vi "SHG_polarization_resolved.vi"() -> ()   [LabVIEW 2022 SP3]
uses:
  PMT_VIs/Logo.ctl
  C:/Users/Public/OneDrive/Desktop/PMT_Project_folder/Kinesis_VIs/Thorlabs.MotionControl.Controls.dll
  Kinesis_VIs/Thorlabs.MotionControl.Controls.dll
  <vilib>/Utility/file.llb/Write Delimited Spreadsheet (string).vi
  <vilib>/Utility/file.llb/Write Delimited Spreadsheet (I64).vi
  <vilib>/Utility/file.llb/Write Delimited Spreadsheet (DBL).vi
  C:/Users/Public/OneDrive/Desktop/PMT_Project_folder/Kinesis_VIs/ThorLabs.MotionControl.KCube.DCServoCLI.dll
  Kinesis_VIs/ThorLabs.MotionControl.KCube.DCServoCLI.dll
  <vilib>/Analysis/NI_AALBase.lvlib
panel:
  in  "Rotating":dbl(ring)=2.0 items=["Analyzer"=1.0, "Polarizer"=2.0, ""=0.0]
  in  "Analyzer config":string="165"
  in  "Polarizer config":string=" rotate"
  in  "autosweep file to save":path=path "D:/LabData/XiaoWang_Group_data_2024on/StackingTransitions/NbOI2/Lvgroup/samples/22p5deg/SHG/flake2_pos1_analyzer-y.txt"
  in  "SP 2":dbl=-5.0 caption="Second Polarizer Start Position \n Set"
  out "SPD 2":dbl=-5.0 caption="Analyzer Start Position Read"
  in  "second motor T/F":bool
  out "PC 2":dbl caption="Second Polarizer Current Position"
  in  "Motor Controller\nSerialNumber 2":string="27261255"
  in  "KCubeDCServoControl 2":refnum<k24>(container)
  out "Polar Plot":picture
  in  "Wait to Start (ms)":i32
  in  "Laser Power (mW)":string="3"
  in  "Sample Name":string="NbOI2 22.5deg flake2 pos1 analyzer-y"
  in  "Save All Gate Data":bool
  out "ESD":dbl caption="Steps\nAdded/Removed"
  in  "ES":dbl caption="Add /Remove \nSteps"
  out "Sweep Graph":u32[](graph)=[236, 252, 257, 253, 238, 214, 204, 173, 152, 146, 141, 143, 145, 162, 179, 184, 196, 197, 202, 190, 177, 161, 155, 148, 142, 151, 152, 169, 188, 216, 224, 233, 239, 236, 224, 211, 194, 170, 151, 147, 143, 143, 157, 168, 177, 196, 198, 205, 196, 190, 170, 163, 146, 136, 133, 134, 144, 165, 186, 211, 229]
  out "SM":i32 caption="Sweep\nMean"
  out "SN":i32=61 caption="Current Sweep Iteration"
  out "SND":i32=61 caption="Total No. of Sweeps"
  in  "Auto-Sweep":bool
  in  "P8":bool
  out "PC":dbl caption="Current Position"
  out "WTD":i32=2500 caption="Wait Time \n(ms) Read"
  out "EPD":dbl=183.0 caption="End Position\nRead"
  out "SPD":dbl caption="Start Position\nRead"
  out "SSD":dbl=3.0 caption="Step Size\nRead"
  in  "SP":dbl caption="Start Position Set"
  in  "WT":i32=2500 caption="Wait Time (ms)\n Set"
  in  "EP":dbl=183.0 caption="End Position Set"
  in  "P7":bool
  in  "SS":dbl=3.0 caption="Step Size Set"
  in  "Motor Controller\nSerialNumber":string="27268499"
  in  "KCubeDCServoControl":refnum<k24>(container)
  in  "Export":bool
  out "DB":u32[](array[numeric])=[235, 0, 0, 0, 0, 0, 0, 0, 0, 0, 0, 0, 0, 0, 0, 0]
  out "OVL":bool caption="LED ON : Over Rang Data"
  out "OLD":i32
  out "GN":i32 caption="Gate Number"
  in  "Correction":bool=TRUE
  in  "Logo":T1
  out "Graph":u32[](graph)=[235]
  in  "Stop":bool
  in  "Start":bool
  in  "P6":bool
  out "RND":i32=20 caption="Read Number\nRead Data"
  in  "P5":bool
  in  "RN":i32=20 caption="Read Number\nSet Data"
  out "PowerD":i32=1 caption="Power\nRead Data"
  out "ITD":i32=400 caption="Internal Time\nRead Data"
  in  "P4":bool
  in  "P3":bool
  in  "IT":i32=400 caption="Internal Time\nSet Data"
  in  "P2":bool
  out "Handle Number":i32=172291552
  in  "P1":bool=TRUE caption="Switch\nPower OFF/Power ON"
  in  "EXIT":bool=TRUE
  # "pmt serial: 30430219"
  # "can't change after running. exit to change"
  # "number in degrees."
  # "y-165\nx-75"
  # "y-82.5\nx-37.5"
  # "polarizer: 27268499\nanalyzer: 2726155"
  # "note: If you change angle between linear polarized light and half-wave plate by theta, the \npolarization after the wave plate is changed by twice theta. The code doesn't account for this.\nThis means we really need to go only to 180degrees, because at that point we have rotated the polarization by 360deg."
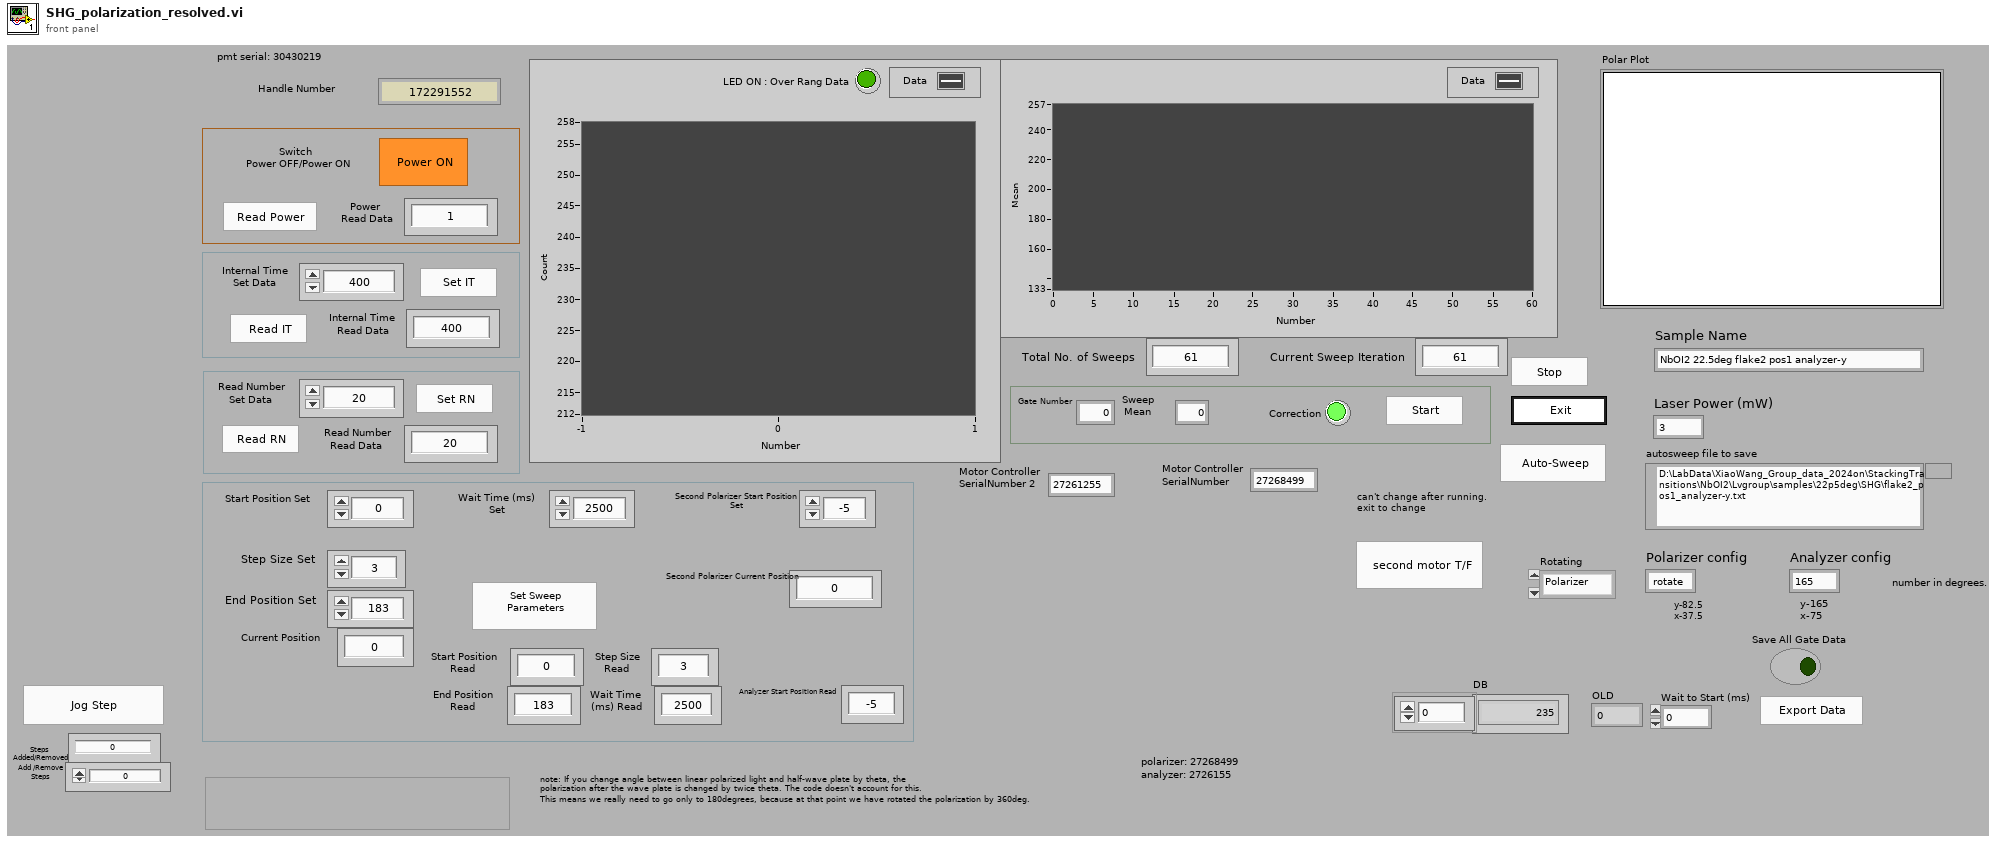
[diagram p1: front panel]
types:
  T1 = typedef "Logo.ctl" = bool
  T2 = enum8{"Enabled", "Disabled", "Disabled and Grayed Out"}
  T3 = typedef "LVBoundsTypeDef.ctl" = cluster{"Width":u32, "Height":u32}
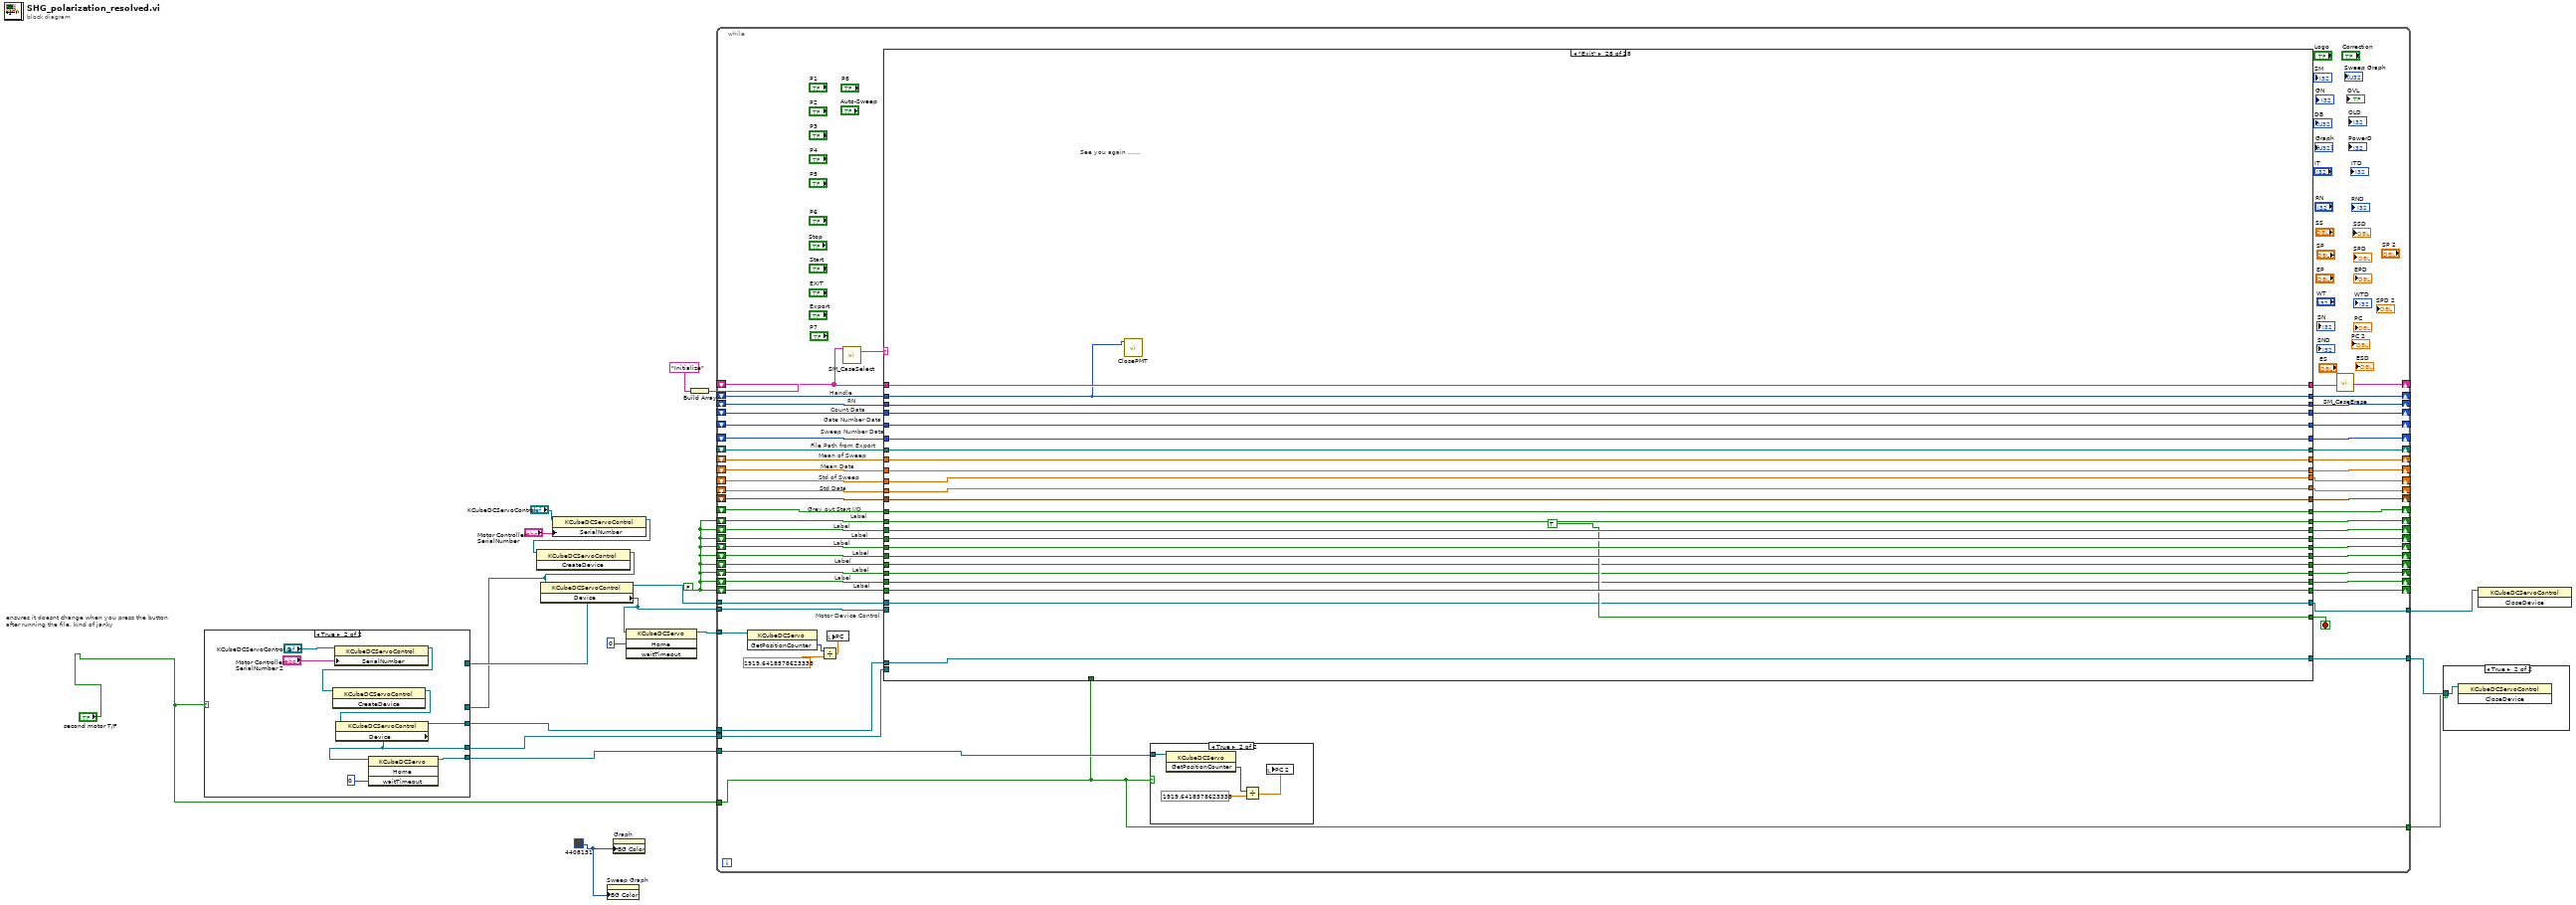
[diagram p0: block diagram]
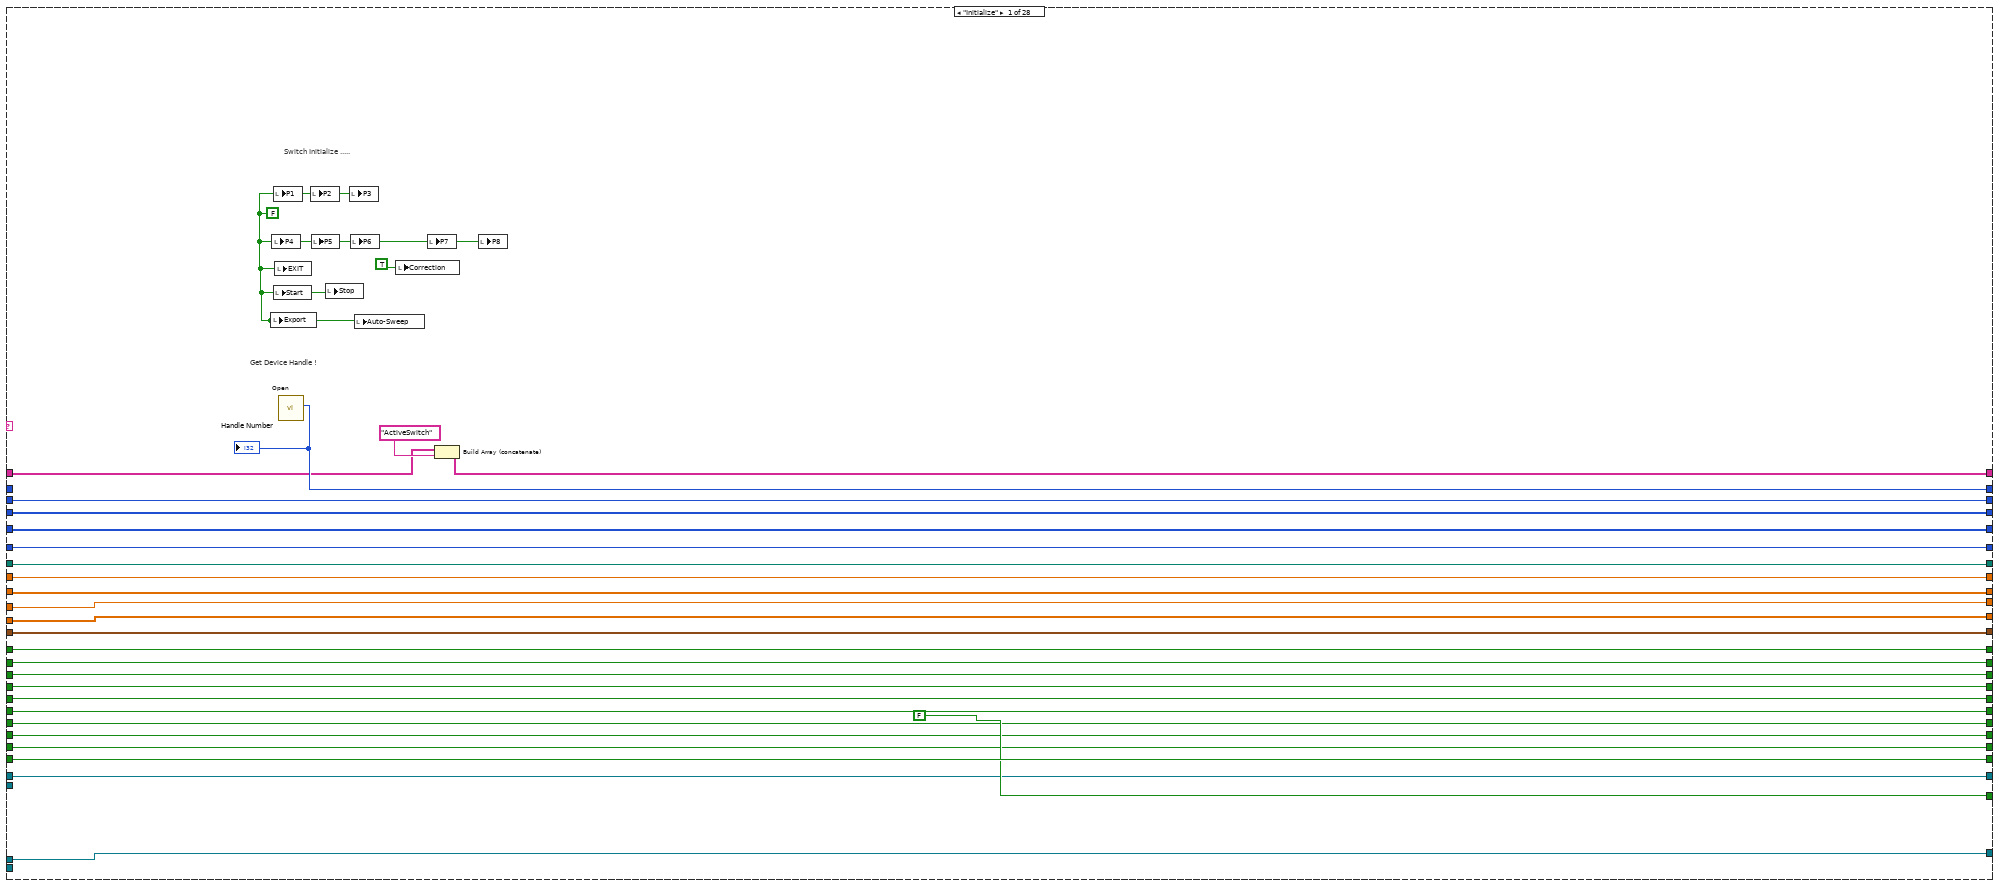
[diagram p5: hidden frame]
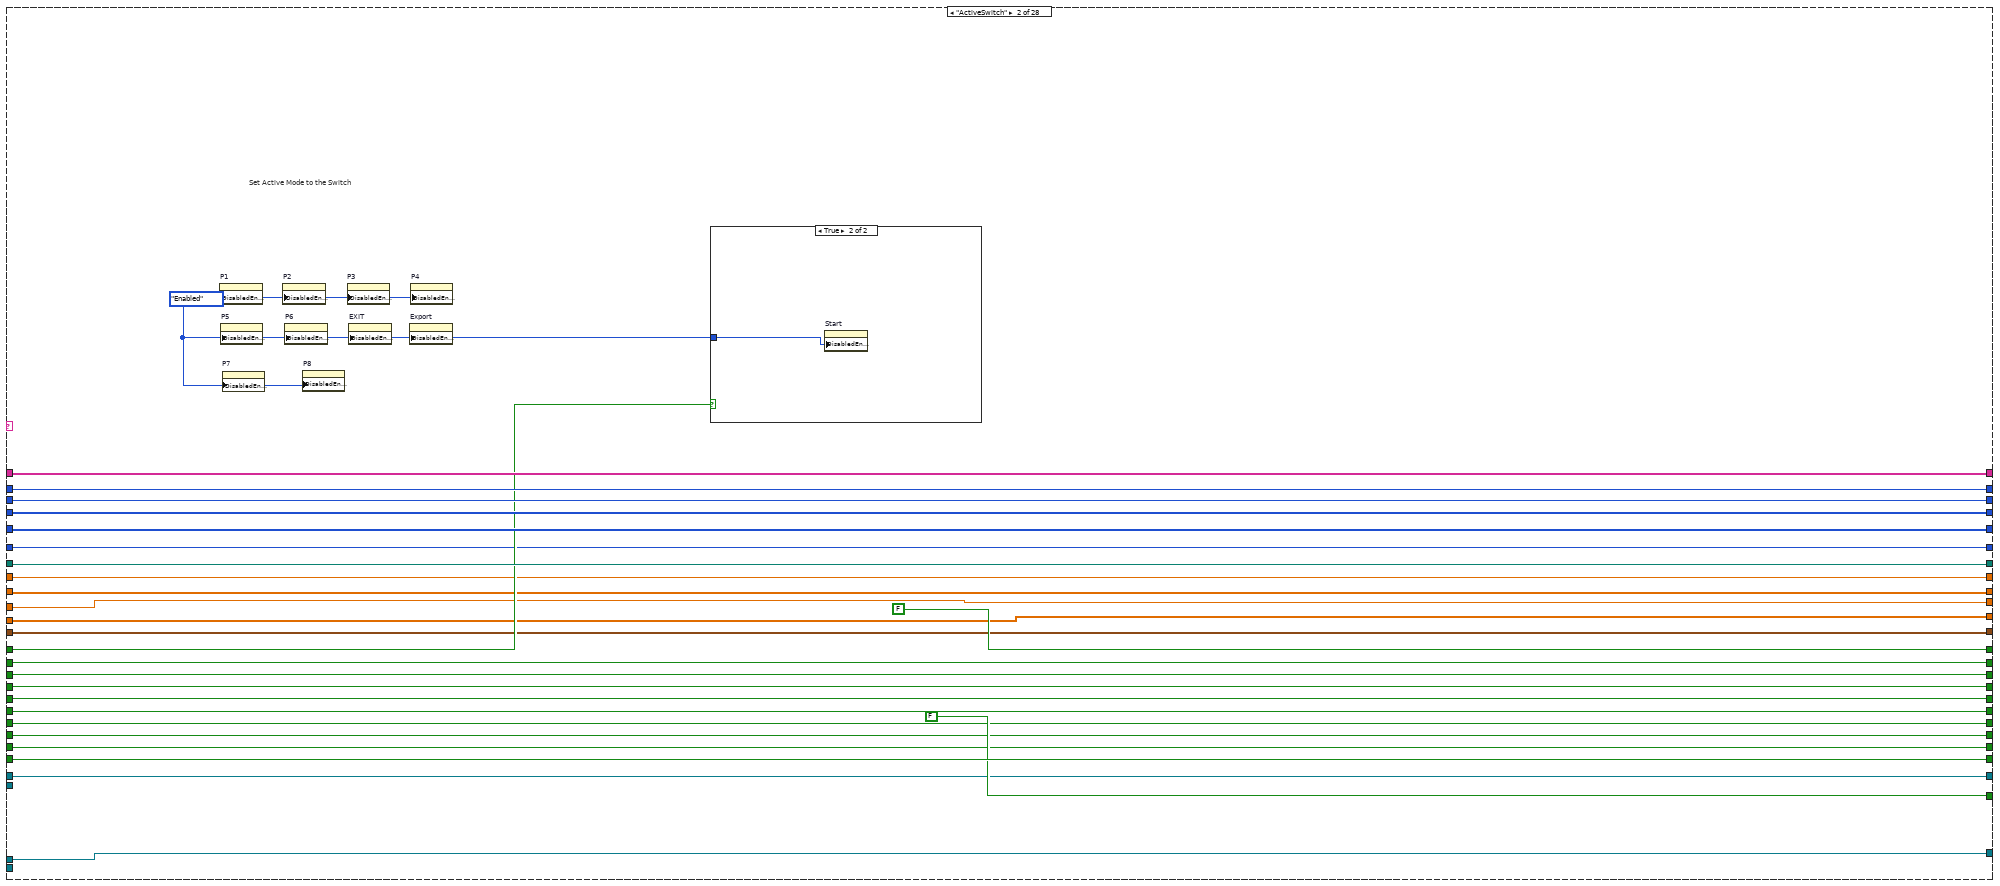
[diagram p6: hidden frame]
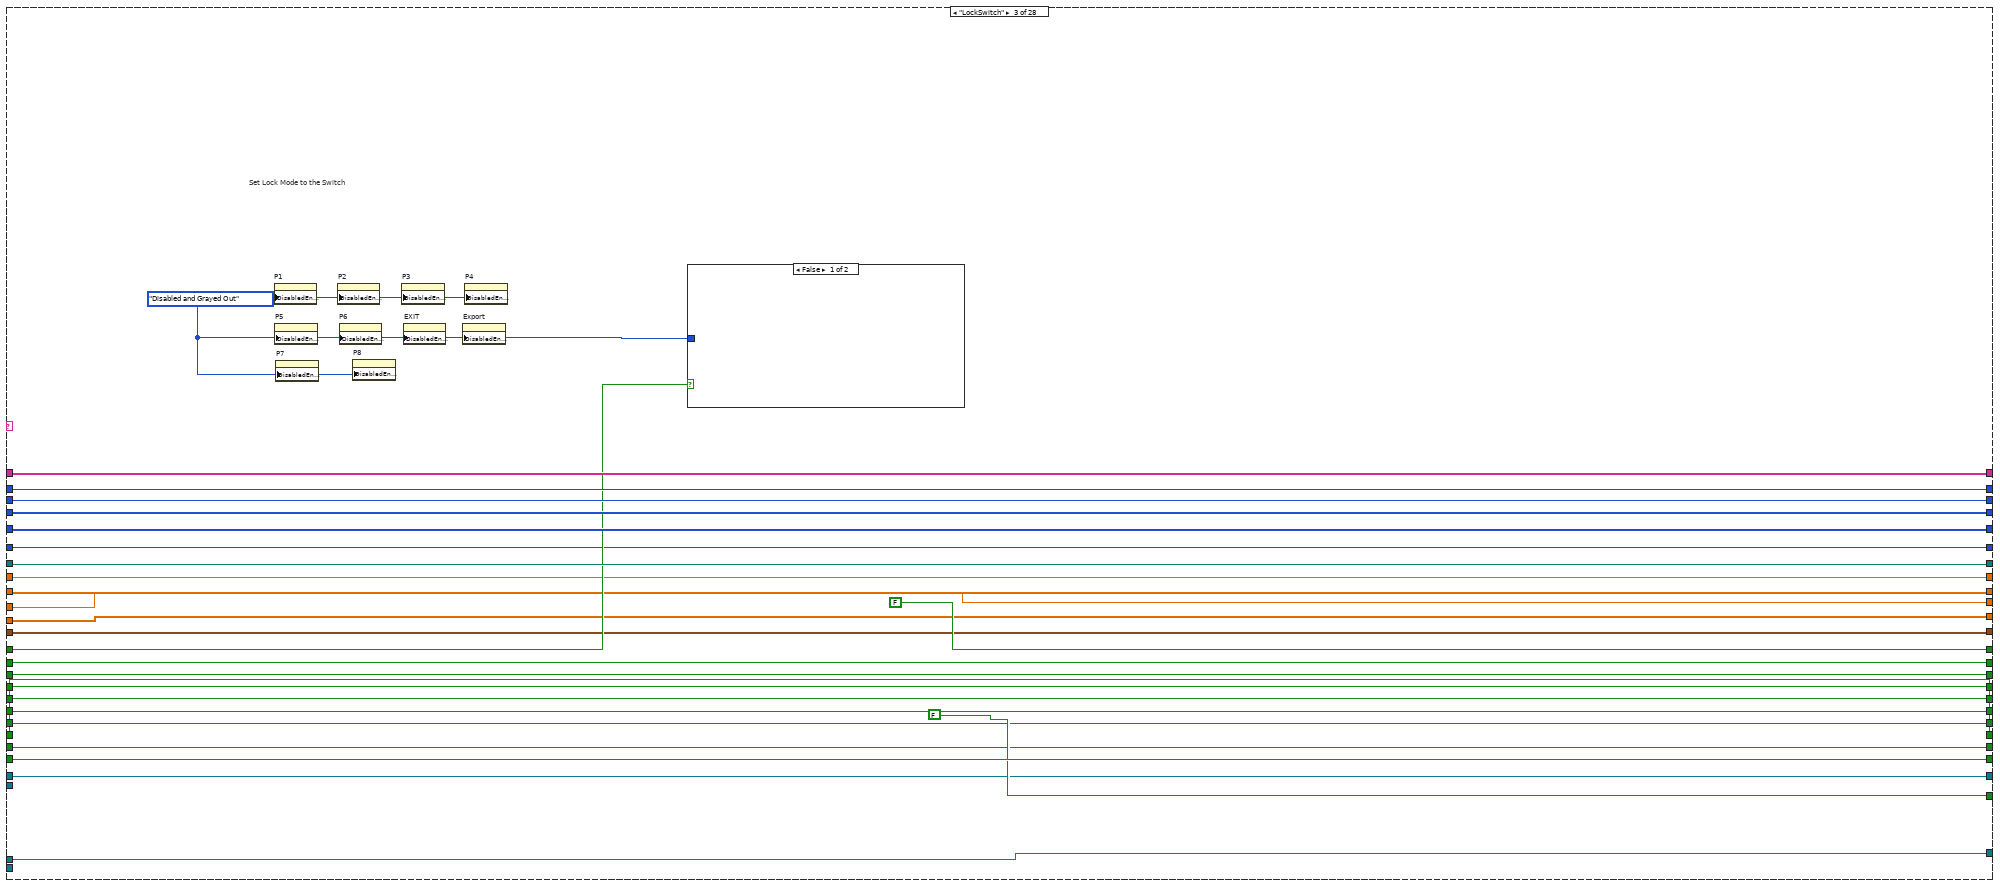
[diagram p8: hidden frame]
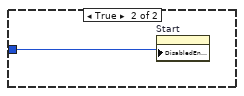
[diagram p9: hidden frame]
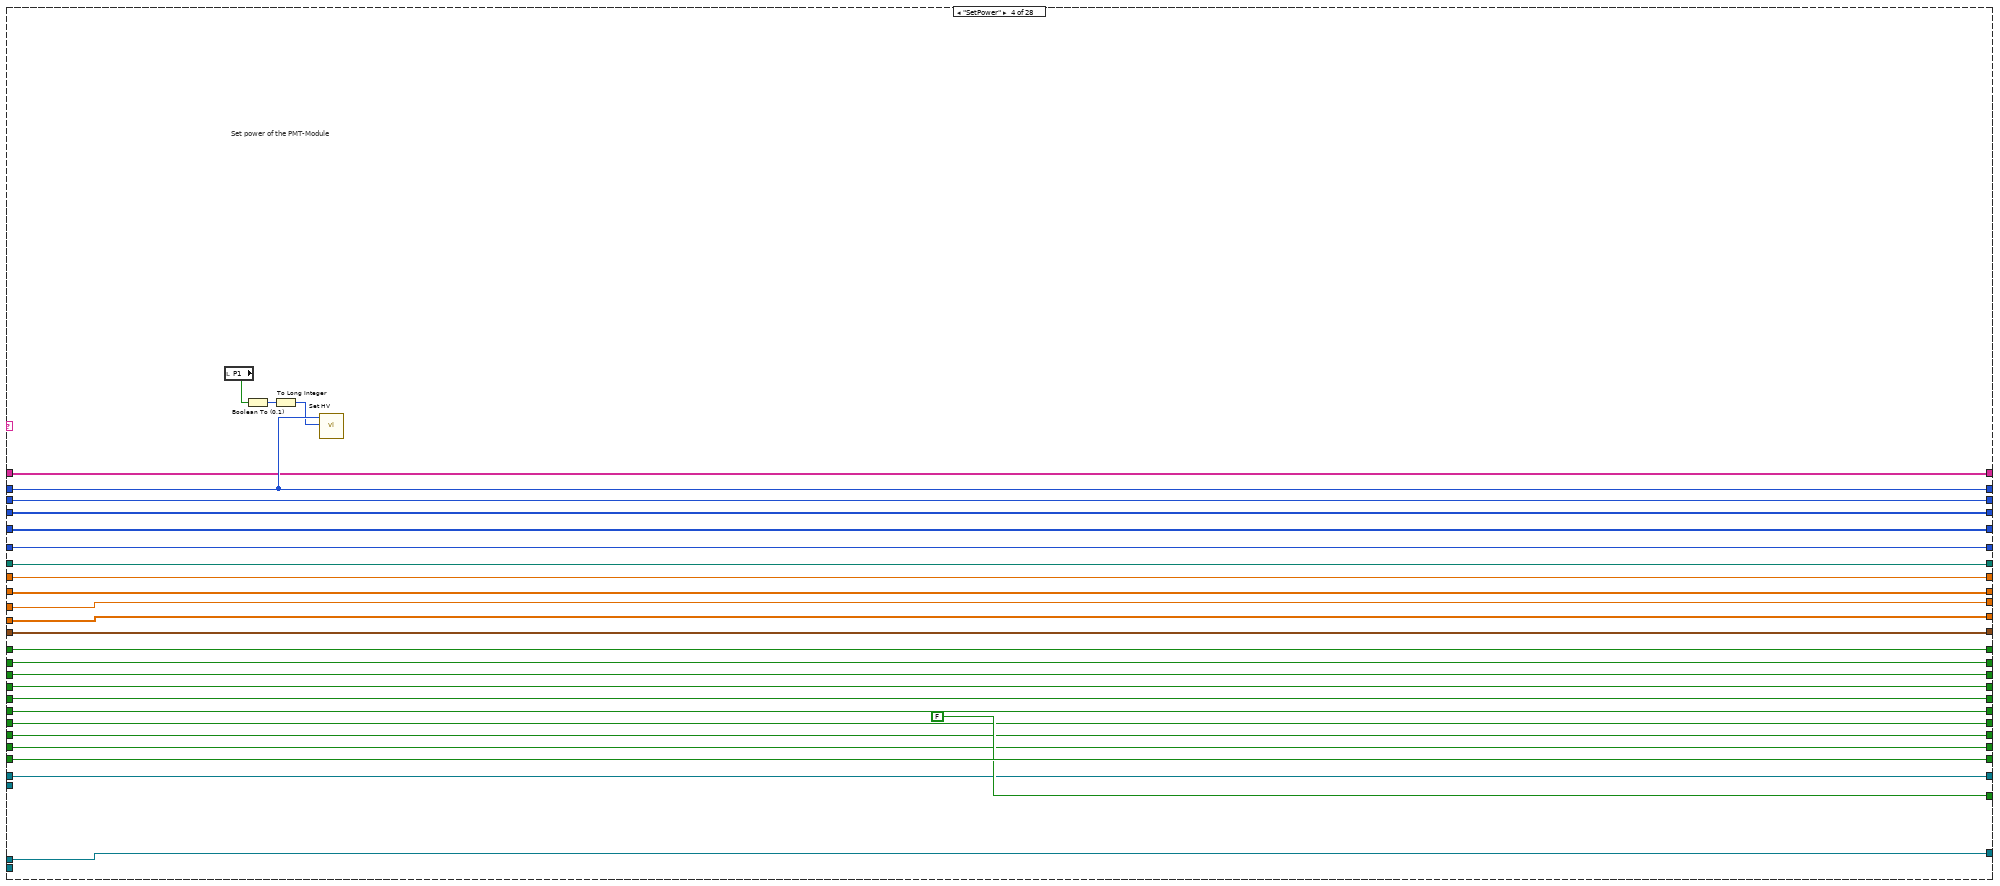
[diagram p10: hidden frame]
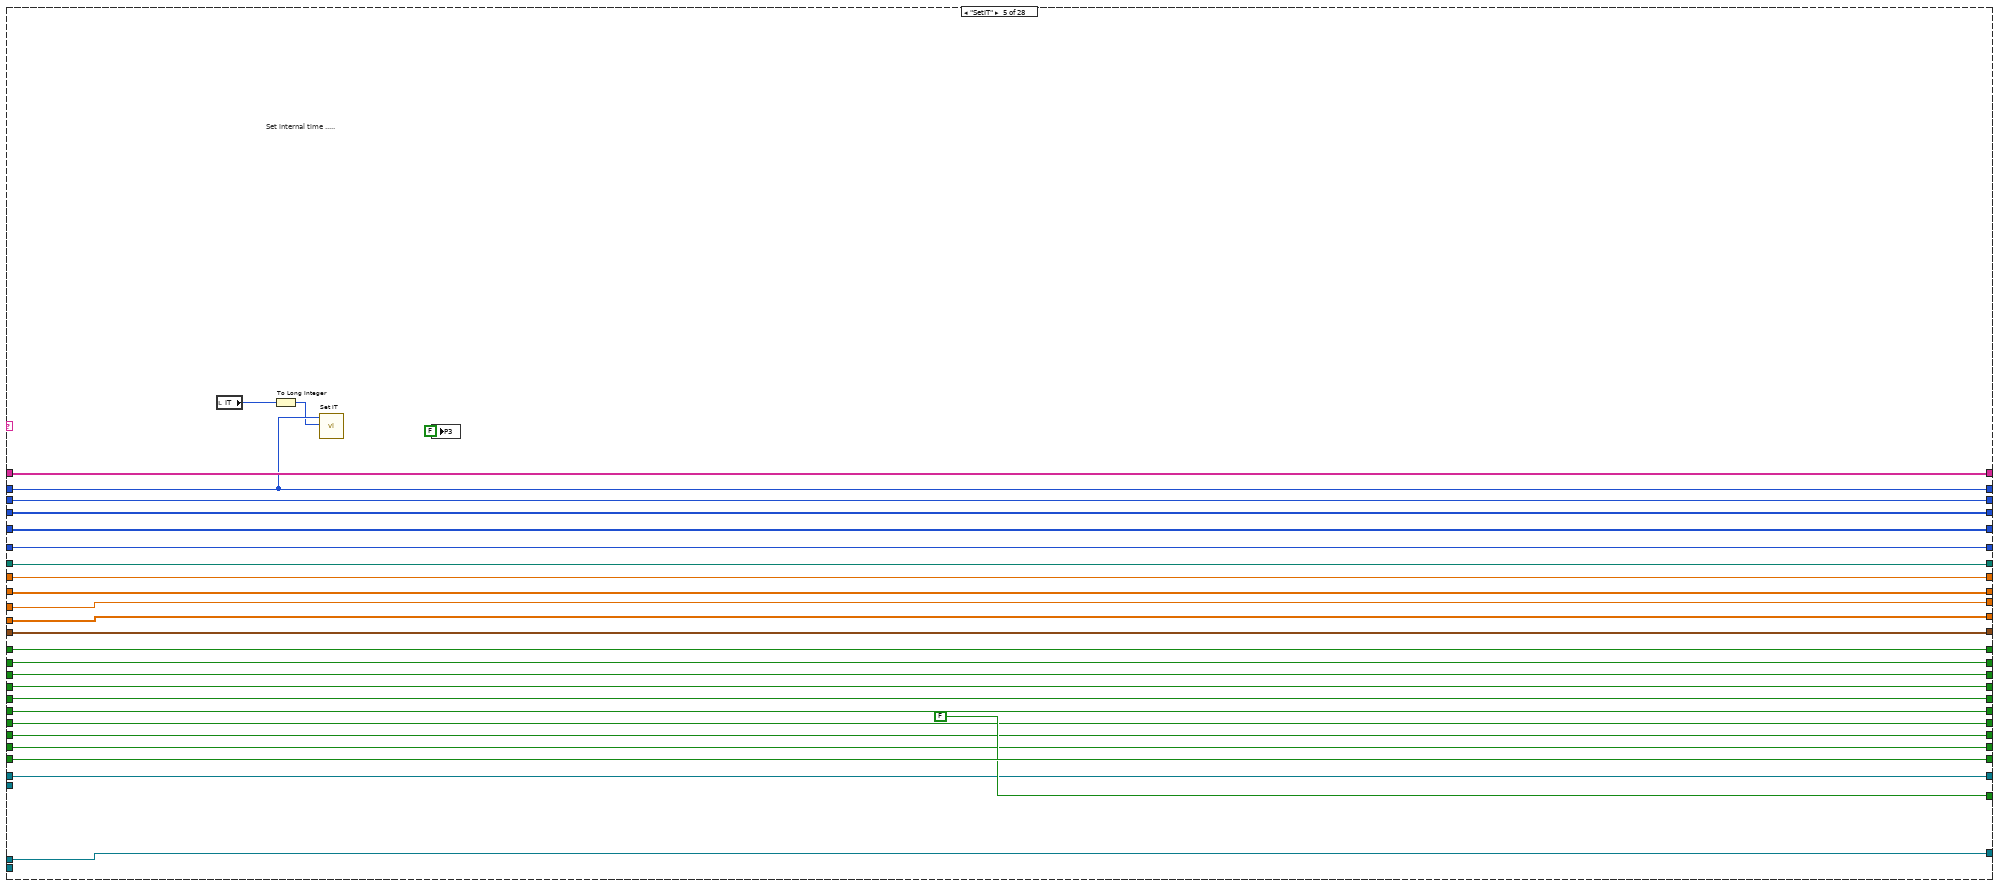
[diagram p11: hidden frame]
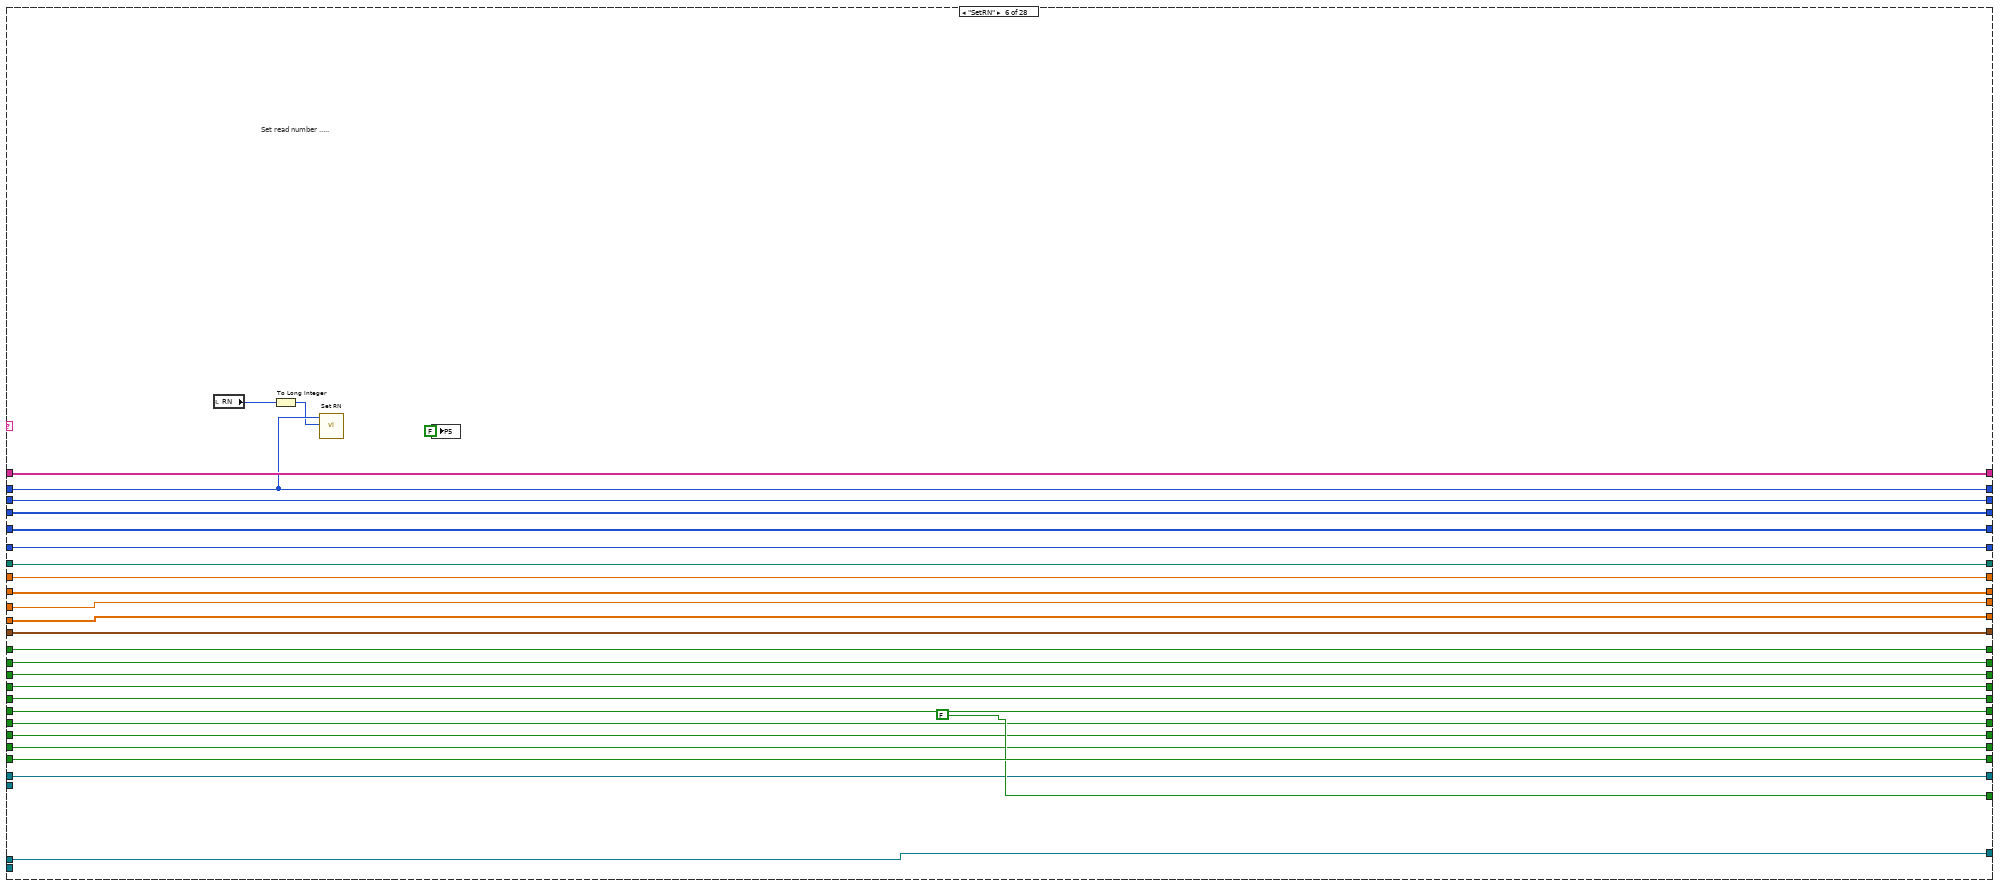
[diagram p12: hidden frame]
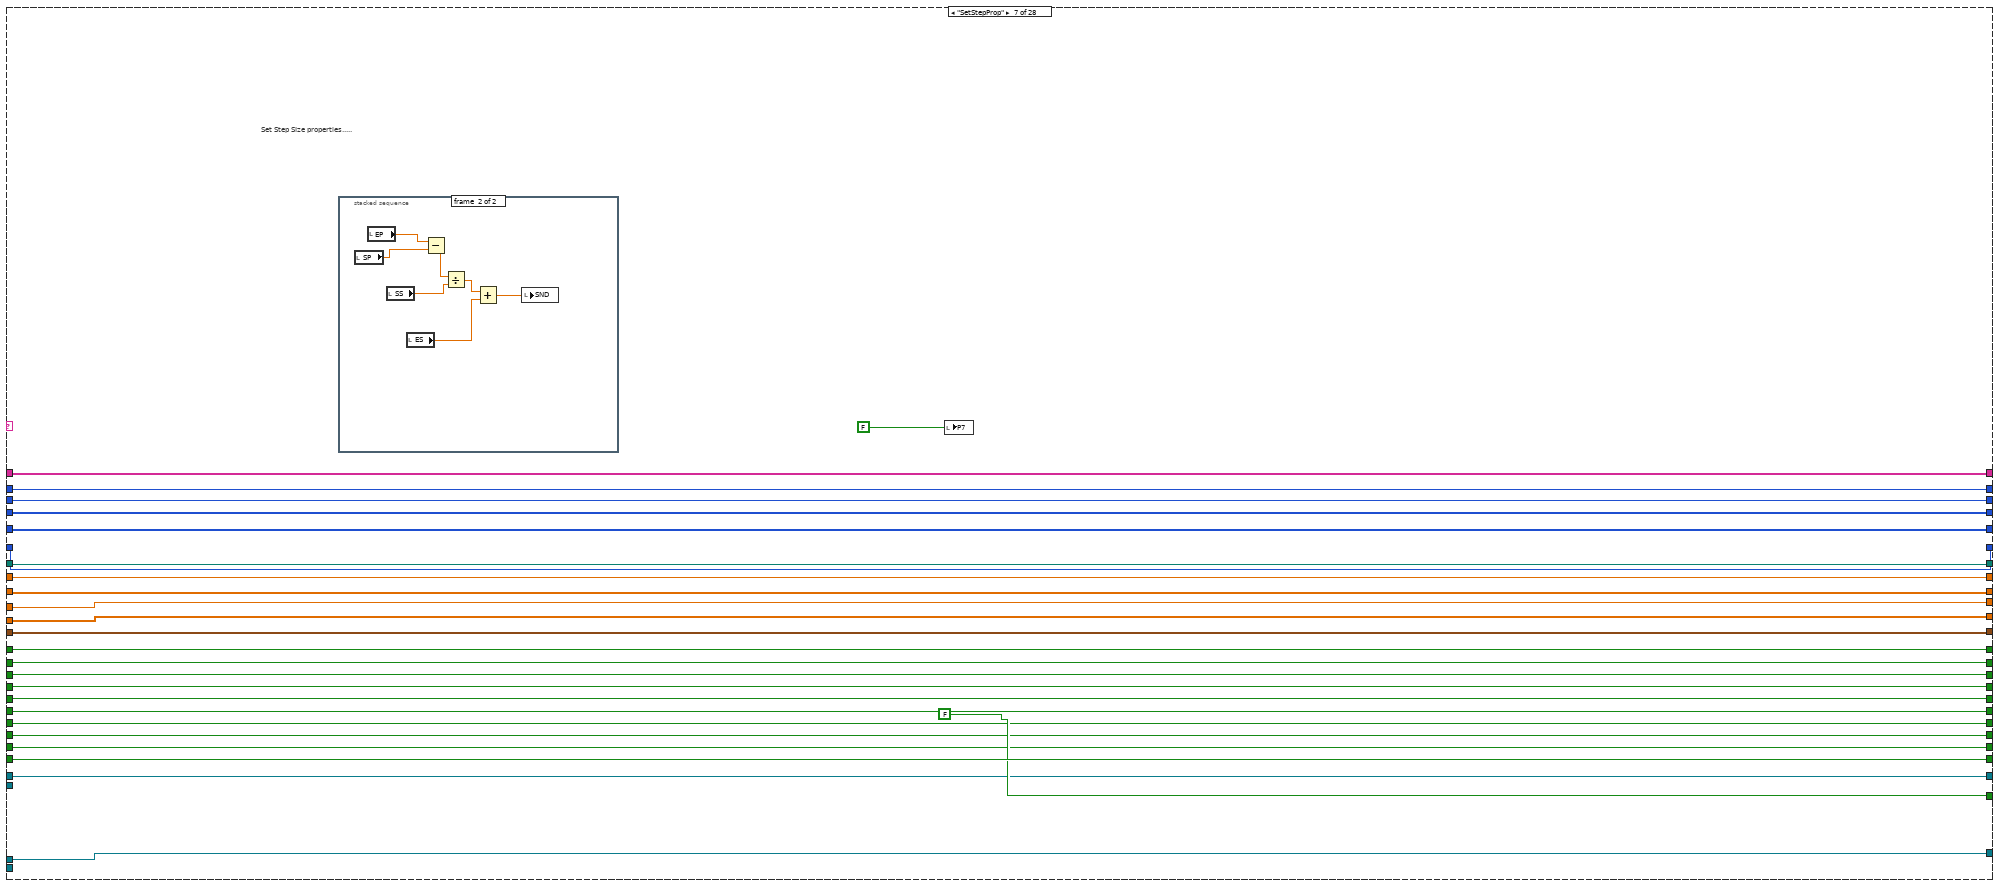
[diagram p13: hidden frame]
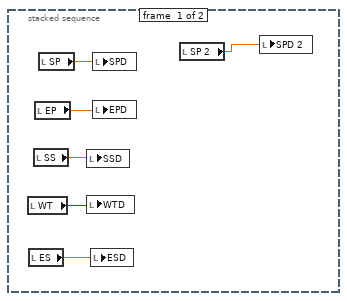
[diagram p14: hidden frame]
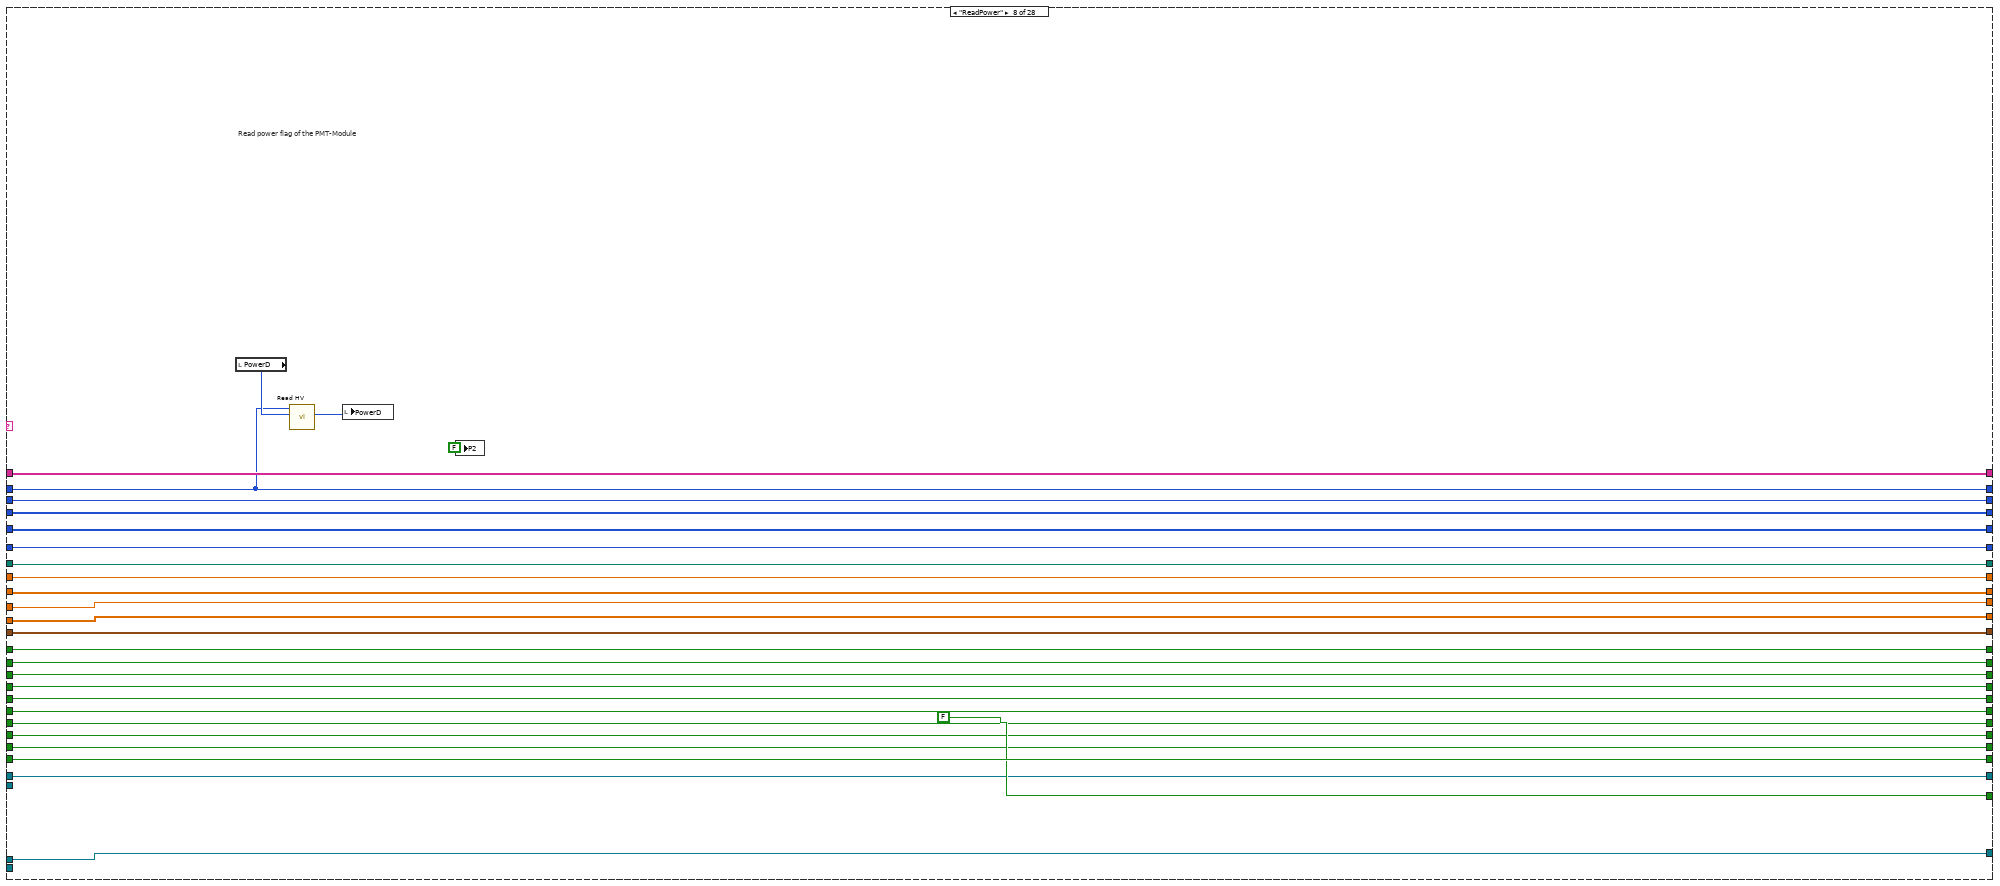
[diagram p15: hidden frame]
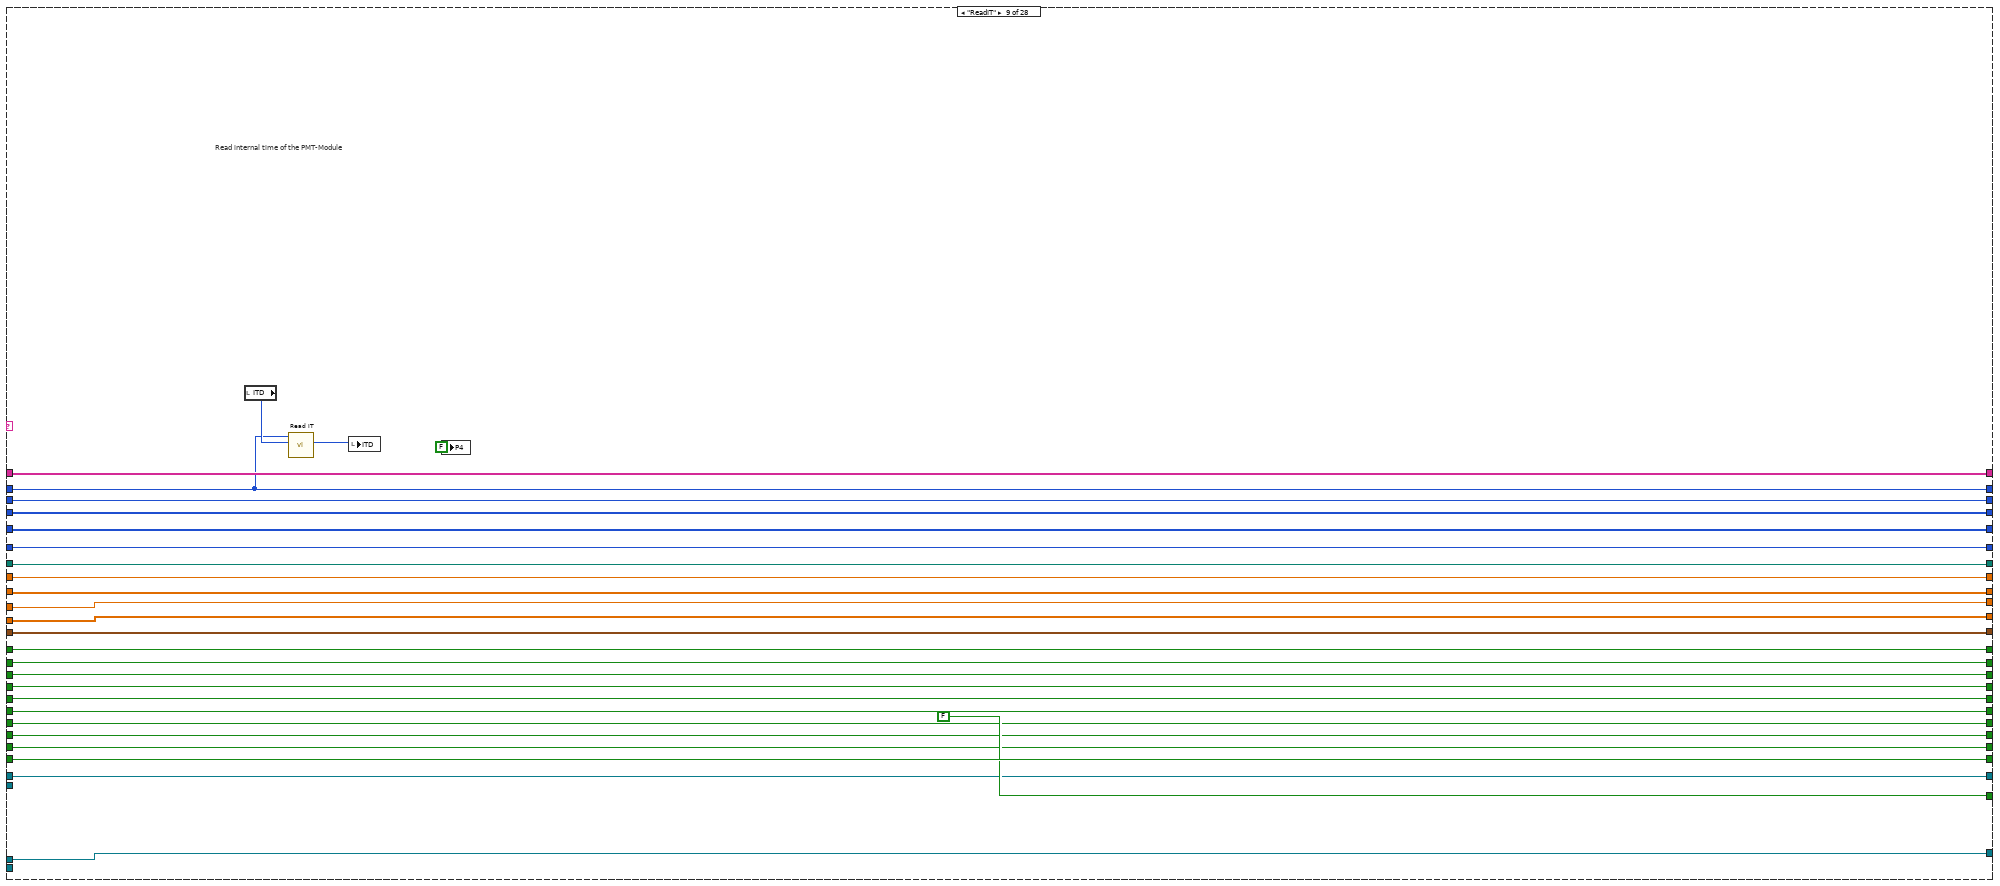
[diagram p16: hidden frame]
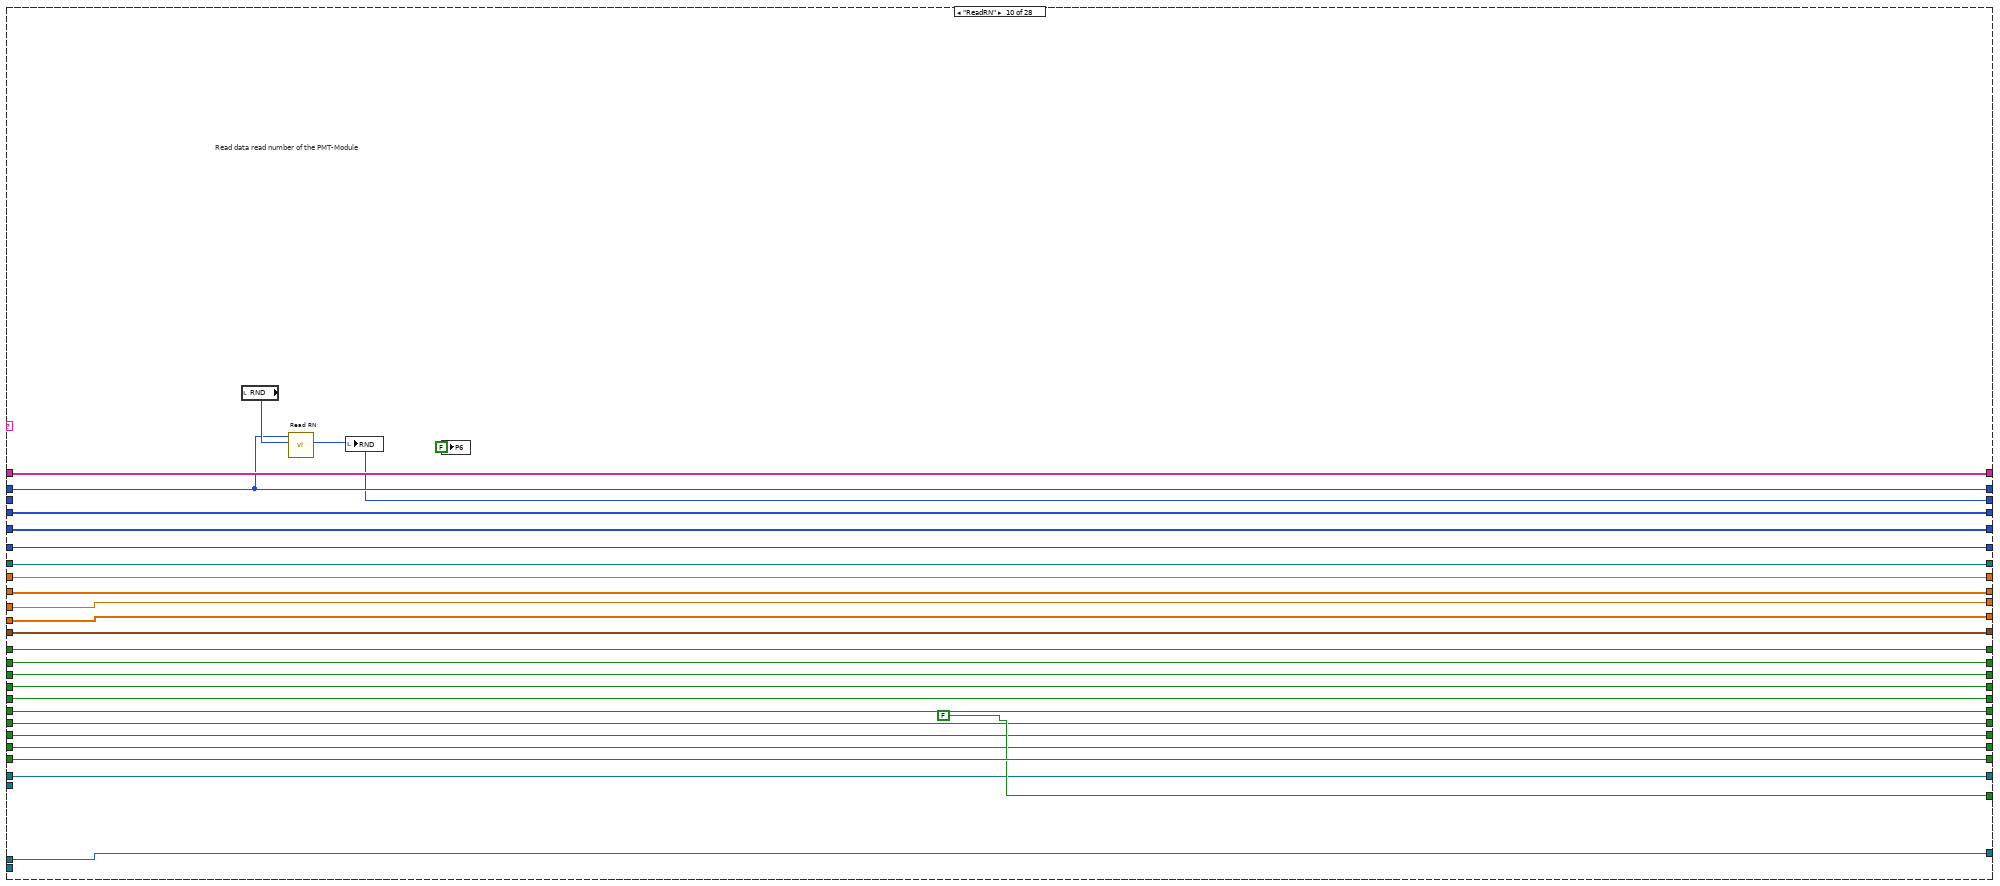
[diagram p17: hidden frame]
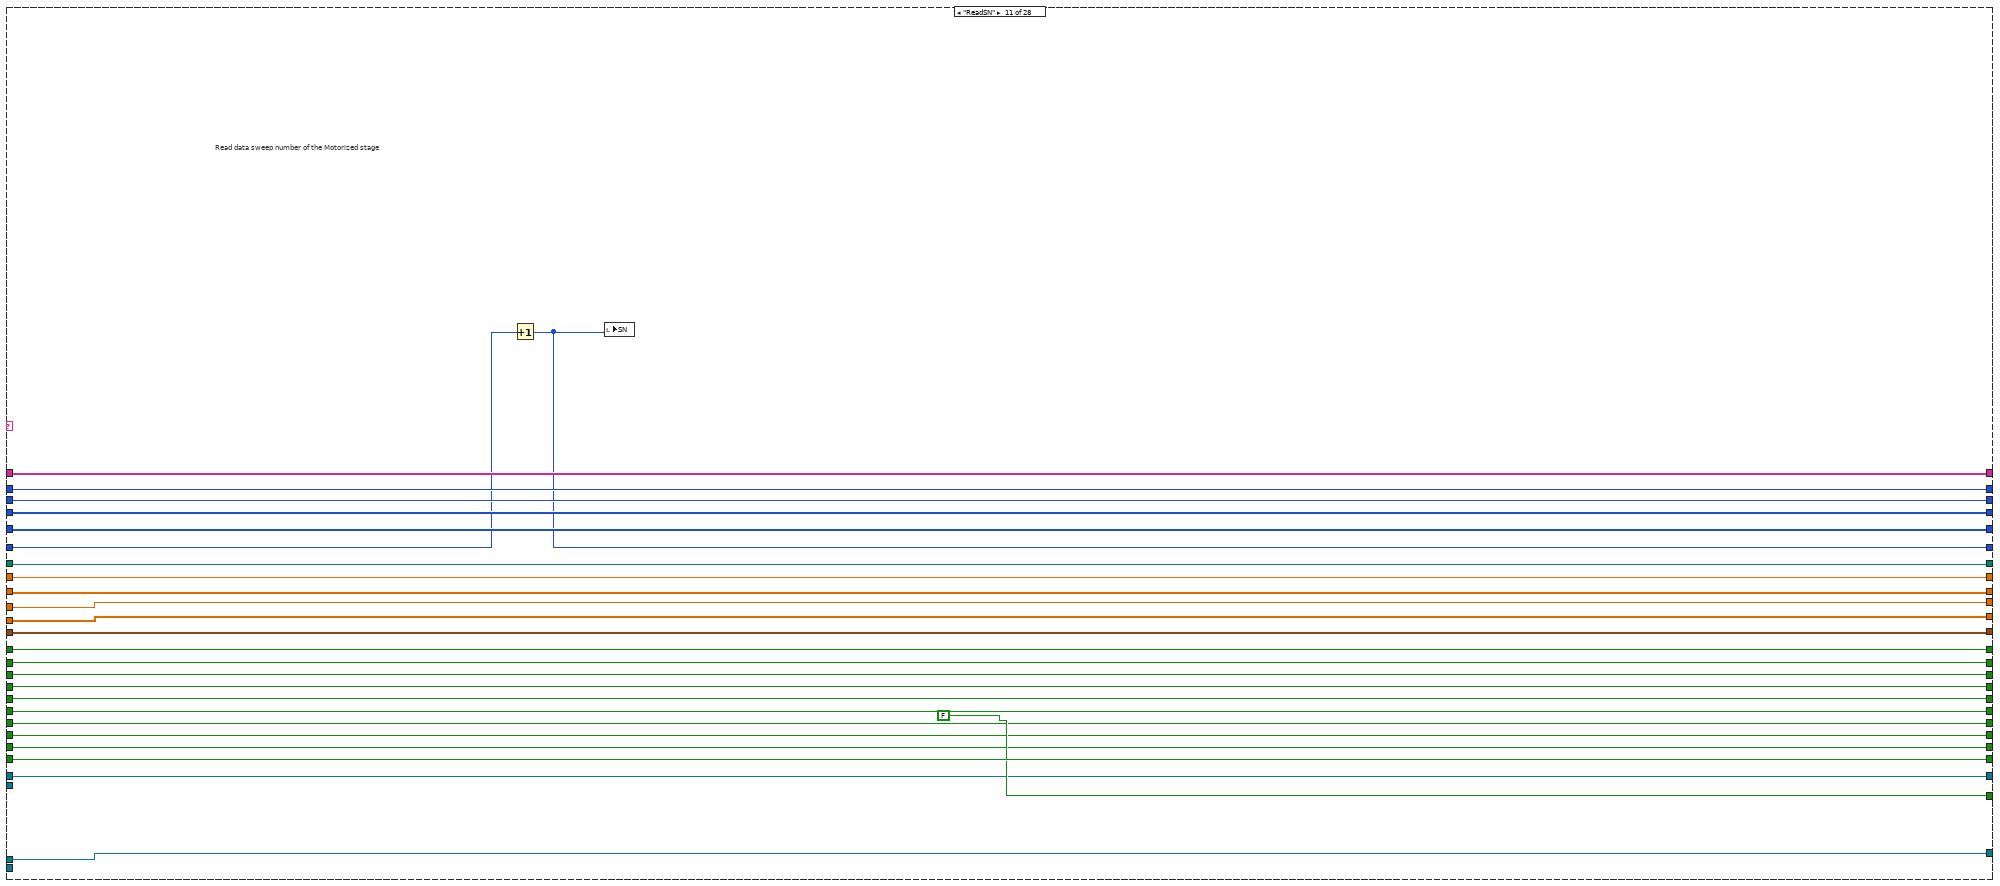
[diagram p18: hidden frame]
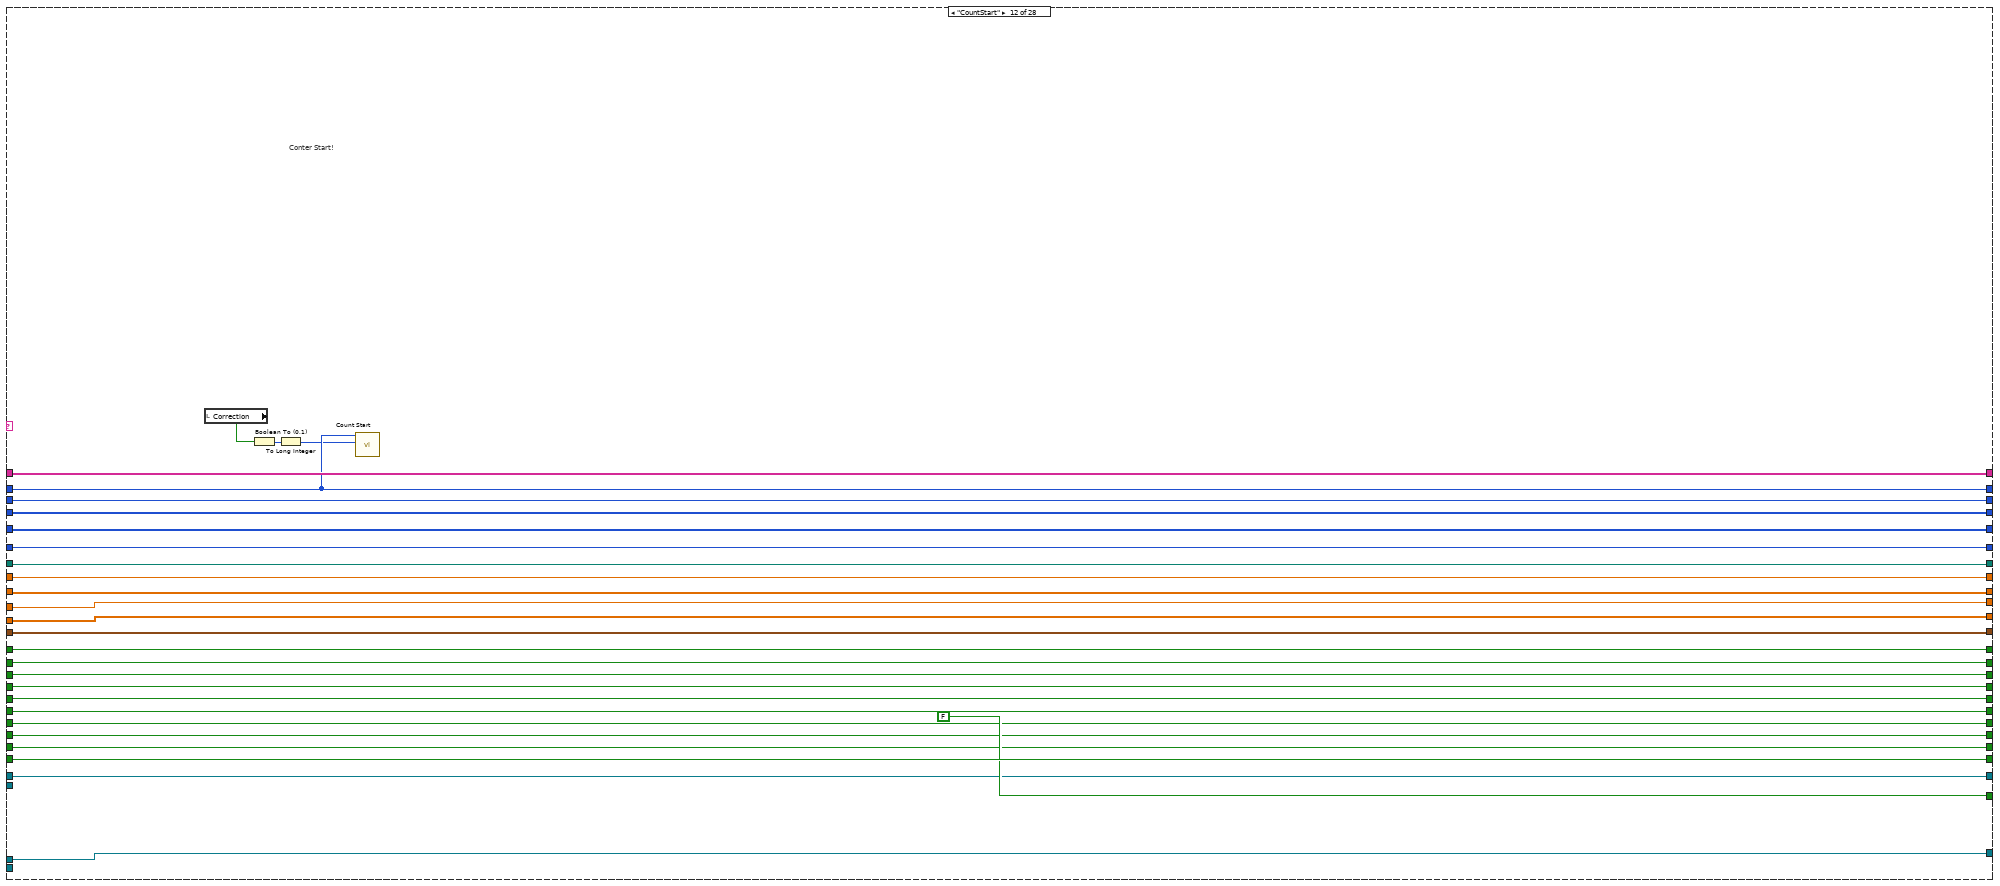
[diagram p19: hidden frame]
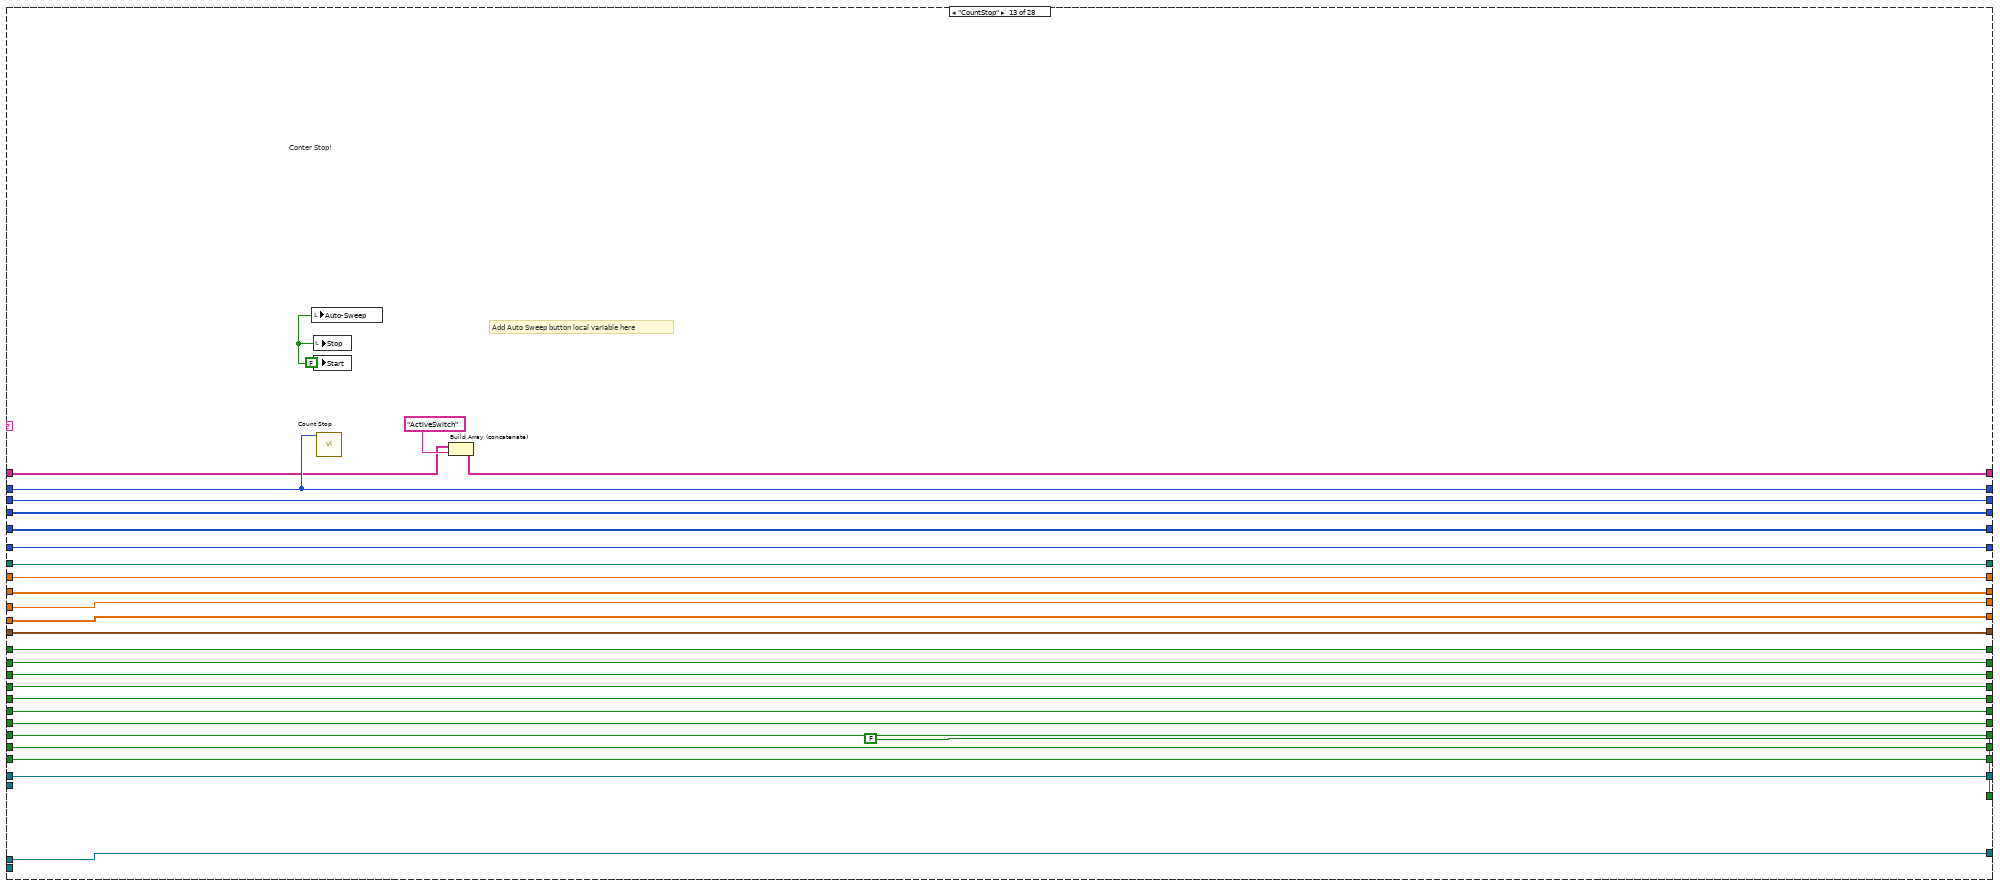
[diagram p20: hidden frame]
diagram:
  w1 = u32 4408131
  w17 = FALSE
  # "ensures it doesnt change when you press the button \nafter running the file. kind of janky"
  n1 = property class="KCubeDCServoControl"(reference="KCubeDCServoControl", "SerialNumber"="Motor Controller\nSerialNumber") -> (reference out=w16:refnum<k24>)  [unwired: 1 in, 1 out]
  n2 = invoke class="KCubeDCServoControl" method="CreateDevice"(reference=w16) -> (reference out=w4:refnum<k24>)  [unwired: 2 in, 2 out]
  n3 = property class="KCubeDCServoControl"(reference=w4) -> (reference out=w13:refnum<k24>, "Device"=w5:refnum<k24>)  [unwired: 1 in, 1 out]
  n4 = case shown="True" "second motor T/F" {
    tunnel: [w20 w24] -> w9
    tunnel: [w20 w23] -> w8
    tunnel: [w21 w22] -> w7
    tunnel: w5 -> [w20 _]
    tunnel: w4 -> [w21 _]
    frame False {
      # "just connect to the first one. it won't be sused"
    }
    frame True {
      n5 = property class="KCubeDCServoControl"(reference="KCubeDCServoControl 2", "SerialNumber"="Motor Controller\nSerialNumber 2") -> (reference out=w29:refnum<k24>)  [unwired: 1 in, 1 out]
      n6 = invoke class="KCubeDCServoControl" method="CreateDevice"(reference=w29) -> (reference out=w26:refnum<k24>)  [unwired: 2 in, 2 out]
      n7 = property class="KCubeDCServoControl"(reference=w26) -> (reference out=w22:refnum<k24>, "Device"=w23:refnum<k24>)  [unwired: 1 in, 1 out]
      n8 = invoke class="KCubeDCServo" method="Home"(reference=w23, "waitTimeout"=0) -> (reference out=w24:refnum<k24>)  [unwired: 2 in, 3 out]
    }
  }
  n9 = property on="Sweep Graph" class="WFGraph (strict)"("BG Color"=w1) -> ()  [unwired: 2 in, 2 out]
  n10 = property on="Graph" class="WFGraph (strict)"("BG Color"=w1) -> ()  [unwired: 2 in, 2 out]
  n11 = invoke class="KCubeDCServo" method="Home"(reference=w5, "waitTimeout"=0) -> (reference out=w11:refnum<k24>)  [unwired: 2 in, 3 out]
  n12 = Build Array("Initialize") -> (w18:string[])
  n13 = while {
    shift-right: [w71] -> _
    shift-left: w17 -> [w72]
    shift-right: [w73] -> _
    shift-left: w17 -> [w74]
    shift-right: [w75] -> _
    shift-left: w17 -> [w76]
    shift-right: [w77] -> _
    shift-left: w17 -> [w78]
    shift-right: [w79] -> _
    shift-left: _ -> [w80]
    shift-right: [w81] -> _
    shift-left: _ -> [w82]
    shift-right: [w83] -> _
    shift-left: _ -> [w84]
    shift-right: [w69] -> _
    shift-left: w17 -> [w70]
    shift-right: [w87] -> _
    shift-left: w17 -> [w88]
    shift-right: [w66] -> _
    shift-left: w18 -> [w85]
    shift-right: [w64] -> _
    shift-left: w17 -> [w65]
    shift-right: [w62] -> _
    shift-left: w17 -> [w63]
    shift-right: [w61] -> _
    shift-left: w17 -> [w60]
    tunnel: w13 -> [w57]
    tunnel: [w56] -> w14
    shift-right: [w59] -> _
    shift-left: _ -> [w58]
    tunnel: w5 -> [w55]
    shift-right: [w54] -> _
    shift-left: _ -> [w53]
    shift-right: [w52] -> _
    shift-left: _ -> [w51]
    tunnel: w11 -> [w50]
    shift-right: [w48] -> _
    shift-left: _ -> [w49]
    shift-right: [w47] -> _
    shift-left: _ -> [w46]
    shift-right: [w45] -> _
    shift-left: _ -> [w44]
    shift-right: [w40] -> _
    shift-left: _ -> [w41]
    shift-right: [w38] -> _
    shift-left: _ -> [w39]
    shift-right: [w36] -> _
    shift-left: _ -> [w35]
    tunnel: w9 -> [w34]
    tunnel: w8 -> [w32]
    tunnel: w7 -> [w33]
    tunnel: [w31] -> w6
    tunnel: "second motor T/F" -> [w30]
    tunnel: [w30] -> w3
    stop <- w68 stop-if-true
    # "Std Data"
    # "Std of Sweep"
    # "Mean Data"
    # "Mean of Sweep"
    # "Sweep Number Data"
    # "Grey out Start I/O"
    # "Motor Device Control"
    # "File Path from Export"
    # "Gate Number Data"
    # "Label"
    # "Label"
    # "Label"
    # "Label"
    # "Label"
    # "Label"
    # "Label"
    # "Label"
    # "Label"
    # "Count Data"
    # "RN"
    # "Handle"
    n14 = invoke class="KCubeDCServo" method="GetPositionCounter"(reference=w50) -> ("GetPositionCounter"=w42:i32)  [unwired: 2 in, 2 out]
    n15 = Divide(x=w42, y=1919.6418578623338) -> (x/y=w37:dbl)
    n16 = local write "PC"(w37) -> ()
    n17 = call "SM_CaseSelect.vi"("Input"=w85) -> ("Case"=w86:string)  [unwired: 10 out]
    n18 = case shown="\"Exit\"" w86 {
      selector: w86 -> [_ _ _ _ _ _ _ _ _ _ _ _ _ _ _ _ _ _ _ _ _ _ _ _ _ _ w1188 _]
      tunnel: w88 -> [w121 w148 w176 w205 w233 w261 w287 w328 w356 w383 w409 w437 w465 w499 w557 w606 w636 w680 w722 w795 w836 w926 w979 w1010 w1066 w1131 w1206 w1231]
      tunnel: [w121 w148 w176 w205 w233 w261 w287 w328 w356 w383 w409 w437 w465 w499 w557 w606 w636 w680 w722 w795 w836 w926 w979 w1010 w1066 w1131 w1206 w1231] -> w87
      tunnel: w85 -> [w107 w147 w175 w180 w232 w260 w286 w327 w355 w382 w408 w436 w451 w498 w556 w594 w614 w667 w710 w806 w847 w937 w971 w1023 w1079 w1119 w1205 w1230]
      tunnel: [w106 w147 w175 w180 w232 w260 w286 w327 w355 w382 w408 w436 w450 w498 w556 w593 w613 w668 w711 w806 w847 w937 w970 w1023 w1079 w1116 w1205 w1230] -> w67
      tunnel: w84 -> [_ w135 w163 w193 w220 w248 w274 w314 w342 w370 w397 w424 w453 w487 w545 w595 w625 w670 w712 w805 w846 w936 w991 w1022 w1078 w1130 w1204 w1207]
      tunnel: [w109 w135 w163 w193 w220 w248 w274 w314 w342 w370 w397 w424 w453 w487 w545 w595 w625 w670 w712 w805 w846 w936 w991 w1022 w1078 w1130 w1204 w1207] -> w83
      tunnel: w82 -> [w120 w146 w174 w204 w231 w259 w285 w326 w354 _ w390 w435 w464 w497 w555 w605 w635 w665 w708 w804 w845 w935 w990 w1021 w1077 w1129 w1203 w1229]
      tunnel: [w120 w146 w174 w204 w231 w259 w285 w326 w354 w368 w390 w435 w464 w497 w555 w605 w635 w665 w708 w804 w845 w935 w990 w1021 w1077 w1129 w1203 w1229] -> w81
      tunnel: w80 -> [w119 w145 w173 w203 w230 w258 w284 w325 w353 w381 w407 w434 w463 w486 w541 _ _ w661 w706 w780 w831 w916 w989 w1020 w1076 w1115 w1202 w1228]
      tunnel: [w119 w145 w173 w203 w230 w258 w284 w325 w353 w381 w407 w434 w463 w485 w541 w585 w623 w661 w706 w780 w831 w916 w989 w1020 w1076 w1115 w1202 w1228] -> w79
      tunnel: w78 -> [w118 w144 w172 w202 w229 w257 w283 w324 w352 w380 w406 w433 w462 w496 w554 w604 w634 w679 w721 w803 w844 w934 w987 w1018 w1074 w1128 w1201 w1227]
      tunnel: [w118 w144 w172 w202 w229 w257 w283 w324 w352 w380 w406 w433 w462 w496 w554 w604 w634 w679 w721 w803 w844 w934 w987 w1018 w1074 w1128 w1201 w1227] -> w77
      tunnel: w76 -> [w117 w143 w171 w201 w228 w256 w282 w323 w351 w379 w405 w432 w461 w495 w553 w603 w633 w678 w720 w802 w843 w933 w986 w1017 w1073 w1127 w1200 w1226]
      tunnel: [w117 w143 w171 w201 w228 w256 w282 w323 w351 w379 w405 w432 w461 w495 w553 w603 w633 w678 w720 w802 w843 w933 w986 w1017 w1073 w1127 w1200 w1226] -> w75
      tunnel: w74 -> [w116 w142 w170 w200 w227 w255 w281 w322 w350 w378 w404 w431 w460 w494 w552 w602 w632 w677 w719 w801 w842 w932 w985 w1016 w1072 w1126 w1199 w1225]
      tunnel: [w116 w142 w170 w200 w227 w255 w281 w322 w350 w378 w404 w431 w460 w494 w552 w602 w632 w677 w719 w801 w842 w932 w985 w1016 w1072 w1126 w1199 w1225] -> w73
      tunnel: w72 -> [w115 w141 w169 w199 w226 w254 w280 w321 w349 w377 w403 w430 w459 w493 w551 w601 w631 w676 w718 w800 w841 w931 w984 w1015 w1071 w1125 w1198 w1224]
      tunnel: [w115 w141 w169 w199 w226 w254 w280 w321 w349 w377 w403 w430 w459 w493 w551 w601 w631 w676 w718 w800 w841 w931 w984 w1015 w1071 w1125 w1198 w1224] -> w71
      tunnel: w70 -> [w114 w140 w168 w198 w225 w253 w279 w320 w348 w376 w402 w429 w458 w492 w550 w600 w630 w675 w717 w799 w840 w930 w983 w1014 w1070 w1124 w1197 w1223]
      tunnel: [w114 w140 w168 w198 w225 w253 w279 w320 w348 w376 w402 w429 w458 w492 w550 w600 w630 w675 w717 w799 w840 w930 w983 w1014 w1070 w1124 w1197 w1223] -> w69
      tunnel: [FALSE FALSE FALSE FALSE FALSE FALSE FALSE FALSE FALSE FALSE FALSE FALSE FALSE FALSE FALSE FALSE FALSE FALSE FALSE FALSE FALSE FALSE FALSE FALSE FALSE FALSE FALSE TRUE] -> w68
      tunnel: w65 -> [w110 w136 w164 w194 w221 w249 w275 w316 w344 w372 w398 w425 w454 w488 w546 w596 w626 w671 w713 w798 w839 w929 w982 w1013 w1069 w1120 w1193 w1219]
      tunnel: [w110 w136 w164 w194 w221 w249 w275 w316 w344 w372 w398 w425 w454 w488 w546 w596 w626 w671 w713 w798 w839 w929 w982 w1013 w1069 w1120 w1193 w1219] -> w64
      tunnel: w63 -> [w112 w138 w166 w196 w223 w251 w277 w318 w346 w374 w400 w427 w456 w490 w548 w598 w628 w673 w715 w797 w838 w928 w981 w1012 w1068 w1122 w1195 w1221]
      tunnel: [w112 w138 w166 w196 w223 w251 w277 w318 w346 w374 w400 w427 w456 w490 w548 w598 w628 w673 w715 w797 w838 w928 w981 w1012 w1068 w1122 w1195 w1221] -> w62
      tunnel: [w111 w137 w165 w195 w222 w250 w276 w317 w345 w373 w399 w426 w455 w489 w547 w597 w627 w672 w714 w796 w837 w927 w980 w1011 w1067 w1121 w1194 w1220] -> w61
      tunnel: w60 -> [w111 w137 w165 w195 w222 w250 w276 w317 w345 w373 w399 w426 w455 w489 w547 w597 w627 w672 w714 w796 w837 w927 w980 w1011 w1067 w1121 w1194 w1220]
      tunnel: [w105 w134 w162 w189 w216 w244 w273 w311 w339 w367 w396 w420 w449 w484 w540 w585 w623 w660 w705 w775 w817 w911 w988 w1019 w1075 w1114 w1187 w1218] -> w59
      tunnel: w58 -> [w105 w134 w162 w189 w216 w244 w273 w311 w339 w367 w396 w420 w449 w483 w540 _ _ w660 w705 w775 w817 w911 w988 w1019 w1075 w1114 w1187 w1218]
      tunnel: w57 -> [w104 w133 w161 w188 w215 w243 w272 w310 w338 w366 w395 w419 w448 w482 w544 w584 w622 w659 w704 w777 w829 w913 w978 w1009 w1065 w1113 w1186 w1217]
      tunnel: [w104 w133 w161 w188 w215 w243 w272 w310 w338 w366 w395 w419 w448 w482 w544 w584 w622 w659 w704 w777 w829 w913 w978 w1009 w1065 w1113 w1186 w1217] -> w56
      tunnel: w55 -> [_ _ _ _ _ _ _ _ _ _ _ _ _ _ _ _ _ _ _ _ _ _ _ w1006 w1062 _ _ _]
      tunnel: [w103 w132 w160 w187 w214 w242 w270 w309 w337 w365 w394 w418 w447 w481 w543 w583 w621 w658 w703 w768 w827 w898 w967 w1007 w1063 w1112 w1185 w1216] -> w54
      tunnel: w53 -> [w103 w132 w160 w187 w214 w242 w270 w309 w337 w365 w394 w418 w447 w481 w543 w583 w621 w658 w703 w768 w823 w897 _ w1007 w1063 w1112 w1185 w1216]
      tunnel: [w102 FALSE FALSE w186 w213 w241 w269 w308 w336 w364 w393 w417 w446 w480 w531 w582 TRUE w657 w702 w770 w826 w910 w976 w1005 w1061 w1111 w1184 w1215] -> w52
      tunnel: w51 -> [w102 w131 w159 w186 w213 w241 w269 w308 w336 w364 w393 w417 w446 w480 w531 w582 _ w657 _ w770 w826 w910 w976 w1005 w1061 w1111 w1184 w1215]
      tunnel: w49 -> [w100 w128 w156 w185 w212 w240 w268 w307 w335 w363 w388 w416 w445 w479 w542 w581 w619 w656 w701 w769 w822 w907 _ w1001 w1060 w1110 w1183 w1214]
      tunnel: [w100 w128 w156 w185 w212 w240 w268 w307 w335 w363 w389 w416 w445 w479 w542 w581 w619 w656 w701 w769 w822 w907 w968 w1001 w1060 w1110 w1183 w1214] -> w48
      tunnel: [w99 w127 w155 w184 w211 w239 w267 w306 w334 w362 w392 w415 w444 w478 w532 w580 w618 w655 w698 w767 w825 w902 w975 w1003 w1059 w1109 w1182 w1213] -> w47
      tunnel: w46 -> [w99 w127 w155 w184 w211 w239 w267 w306 w334 w362 w392 w415 w444 w478 w532 w580 w618 w655 w698 w767 _ w902 w975 w1003 w1059 w1109 w1182 w1213]
      tunnel: [w98 w126 w154 w183 w210 w238 w266 w305 w333 w361 w391 w414 w443 w477 w539 w579 w617 w654 w697 w766 w824 w906 w969 w1002 w1058 w1108 w1181 w1212] -> w45
      tunnel: w44 -> [w98 w126 w154 w183 w210 w238 w266 w305 w333 w361 w391 w414 w443 w477 w538 w579 w617 w654 w697 w766 w824 w908 w969 w1002 w1058 w1108 w1181 w1212]
      tunnel: w41 -> [w97 w125 w153 w182 w209 w237 w265 w304 w332 w360 w387 w413 w441 w476 w537 w578 w610 w653 w695 w765 w816 w904 w965 w1000 w1057 w1107 w1180 w1211]
      tunnel: [w97 w125 w153 w182 w209 w237 w265 w304 w332 w360 w387 w413 w441 w476 w535 w578 w610 w653 w695 w765 w816 w905 w965 w1000 w1057 w1107 w1180 w1211] -> w40
      tunnel: w39 -> [w96 w124 w152 w181 w208 w236 w264 w303 w331 w359 w386 w412 w440 w475 w536 w577 w609 w652 w694 w764 _ w901 w964 w999 w1056 w1106 w1179 w1210]
      tunnel: [w96 w124 w152 w181 w208 w236 w264 w303 w331 w359 w386 w412 w440 w475 w536 w577 w609 w652 w694 w764 w815 w901 w964 w999 w1056 w1106 w1179 w1210] -> w38
      tunnel: [w94 w123 w151 w179 w207 w235 w263 w302 w330 w358 w385 w411 w439 w474 w529 w576 w608 w651 w693 w763 w813 w888 w962 w998 w1055 w1105 w1178 w1209] -> w36
      tunnel: w35 -> [w94 w123 w151 w179 w207 w235 w263 w302 w330 w358 w385 w411 w439 w474 w530 w576 w608 w651 w693 w763 w813 _ w962 w998 w1055 w1105 w1178 w1209]
      tunnel: w33 -> [w93 w122 w150 w178 w206 w234 w262 w301 w329 w357 w384 w410 w438 w473 w528 w575 w607 w650 w692 w762 w812 w886 w961 w997 w1054 w1104 w1177 w1208]
      tunnel: w32 -> [_ _ _ _ _ _ _ _ _ _ _ _ _ _ _ _ _ _ _ _ _ _ _ w996 w1051 _ _ _]
      tunnel: [w93 w122 w150 w178 w206 w234 w262 w301 w329 w357 w384 w410 w438 w473 w528 w575 w607 w650 w692 w762 w812 w886 w961 w997 w1054 w1104 w1177 w1208] -> w31
      tunnel: w30 -> [_ _ _ _ _ _ _ _ _ _ _ _ _ _ _ _ _ _ _ _ _ _ _ w993 w1048 _ _ _]
      frame "Initialize" {
        w101 = FALSE ("P1")
        # "Get Device Handle !"
        # "Switch Initialize ....."
        n19 = local write "Export"(w101) -> ()
        n20 = local write "P4"(w101) -> ()
        n21 = local write "P1"(w101) -> ()
        n22 = local write "Start"(w101) -> ()
        n23 = local write "EXIT"(w101) -> ()
        n24 = call "Open.vi"() -> ("Handle Number"=w109:i32)  [unwired: 10 in, 1 out]
        "Handle Number" <- w109
        n25 = local write "P2"(w101) -> ()
        n26 = local write "P5"(w101) -> ()
        n27 = local write "Stop"(w101) -> ()
        n28 = local write "P3"(w101) -> ()
        n29 = local write "P6"(w101) -> ()
        n30 = local write "Auto-Sweep"(w101) -> ()
        n31 = local write "Correction"(TRUE ("P1")) -> ()
        n32 = local write "P7"(w101) -> ()
        n33 = Build Array (concatenate)(w107, "ActiveSwitch") -> (w106:string[])
        n34 = local write "P8"(w101) -> ()
      }
      frame "ActiveSwitch" {
        w129 = T2."Enabled" ("無効")
        # "Set Active Mode to the Switch"
        n35 = property on="P1" class="Bool (strict)"("DisabledEnum"=w129) -> ()  [unwired: 2 in, 2 out]
        n36 = property on="P5" class="Bool (strict)"("DisabledEnum"=w129) -> ()  [unwired: 2 in, 2 out]
        n37 = property on="P7" class="Bool (strict)"("DisabledEnum"=w129) -> ()  [unwired: 2 in, 2 out]
        n38 = property on="P2" class="Bool (strict)"("DisabledEnum"=w129) -> ()  [unwired: 2 in, 2 out]
        n39 = property on="P6" class="Bool (strict)"("DisabledEnum"=w129) -> ()  [unwired: 2 in, 2 out]
        n40 = property on="P8" class="Bool (strict)"("DisabledEnum"=w129) -> ()  [unwired: 2 in, 2 out]
        n41 = property on="P3" class="Bool (strict)"("DisabledEnum"=w129) -> ()  [unwired: 2 in, 2 out]
        n42 = property on="EXIT" class="Bool (strict)"("DisabledEnum"=w129) -> ()  [unwired: 2 in, 2 out]
        n43 = property on="Export" class="Bool (strict)"("DisabledEnum"=w129) -> ()  [unwired: 2 in, 2 out]
        n44 = property on="P4" class="Bool (strict)"("DisabledEnum"=w129) -> ()  [unwired: 2 in, 2 out]
        n45 = case shown="True" w131 {
          tunnel: w129 -> [_ w149]
          frame False {
          }
          frame True {
            n46 = property on="Start" class="Bool (strict)"("DisabledEnum"=w149) -> ()  [unwired: 2 in, 2 out]
          }
        }
      }
      frame "LockSwitch" {
        w157 = T2."Disabled and Grayed Out" ("無効")
        # "Set Lock Mode to the Switch"
        n47 = property on="P1" class="Bool (strict)"("DisabledEnum"=w157) -> ()  [unwired: 2 in, 2 out]
        n48 = property on="P5" class="Bool (strict)"("DisabledEnum"=w157) -> ()  [unwired: 2 in, 2 out]
        n49 = property on="P7" class="Bool (strict)"("DisabledEnum"=w157) -> ()  [unwired: 2 in, 2 out]
        n50 = property on="P2" class="Bool (strict)"("DisabledEnum"=w157) -> ()  [unwired: 2 in, 2 out]
        n51 = property on="P6" class="Bool (strict)"("DisabledEnum"=w157) -> ()  [unwired: 2 in, 2 out]
        n52 = property on="P8" class="Bool (strict)"("DisabledEnum"=w157) -> ()  [unwired: 2 in, 2 out]
        n53 = property on="P3" class="Bool (strict)"("DisabledEnum"=w157) -> ()  [unwired: 2 in, 2 out]
        n54 = property on="EXIT" class="Bool (strict)"("DisabledEnum"=w157) -> ()  [unwired: 2 in, 2 out]
        n55 = property on="Export" class="Bool (strict)"("DisabledEnum"=w157) -> ()  [unwired: 2 in, 2 out]
        n56 = property on="P4" class="Bool (strict)"("DisabledEnum"=w157) -> ()  [unwired: 2 in, 2 out]
        n57 = case shown="False" w159 {
          tunnel: w157 -> [_ w177]
          frame False {
          }
          frame True {
            n58 = property on="Start" class="Bool (strict)"("DisabledEnum"=w177) -> ()  [unwired: 2 in, 2 out]
          }
        }
      }
      frame "SetPower" {
        # "Set power of the PMT-Module"
        n59 = local read "P1"() -> (w192:bool)
        n60 = Boolean To (0,1)(Boolean=w192) -> (0, 1=w191:i16)
        n61 = To Long Integer(number=w191) -> (32bit integer=w190:i32)
        n62 = call "Set HV.vi"("HV"=w190, "handle"=w193) -> ()  [unwired: 8 in, 2 out]
      }
      frame "SetIT" {
        # "Set internal time ....."
        n63 = local read "IT"() -> (w218:i32)
        n64 = To Long Integer(number=w218) -> (32bit integer=w219:i32)
        n65 = call "Set IT.vi"("IT"=w219, "handle"=w220) -> ()  [unwired: 8 in, 2 out]
        n66 = local write "P3"(FALSE ("P3")) -> ()
      }
      frame "SetRN" {
        # "Set read number ....."
        n67 = local read "RN"() -> (w246:i32)
        n68 = To Long Integer(number=w246) -> (32bit integer=w247:i32)
        n69 = call "Set RN.vi"("RN"=w247, "handle"=w248) -> ()  [unwired: 8 in, 2 out]
        n70 = local write "P5"(FALSE ("P3")) -> ()
      }
      frame "SetStepProp" {
        # "Set Step SIze properties....."
        n71 = stacked-sequence {
          frame #0 {
            n72 = local read "WT"() -> (w290:i32)
            n73 = local read "ES"() -> (w289:dbl)
            n74 = local read "SS"() -> (w291:dbl)
            n75 = local read "EP"() -> (w292:dbl)
            n76 = local read "SP"() -> (w293:dbl)
            n77 = local write "SSD"(w291) -> ()
            n78 = local write "WTD"(w290) -> ()
            n79 = local write "ESD"(w289) -> ()
            n80 = local write "SPD"(w293) -> ()
            n81 = local write "EPD"(w292) -> ()
            n82 = local read "SP 2"() -> (w288:dbl)
            n83 = local write "SPD 2"(w288) -> ()
          }
          frame #1 {
            n84 = local read "SP"() -> (w294:dbl)
            n85 = local read "EP"() -> (w296:dbl)
            n86 = local read "SS"() -> (w300:dbl)
            n87 = local read "ES"() -> (w298:dbl)
            n88 = Subtract(x=w296, y=w294) -> (x-y=w295:dbl)
            n89 = Divide(x=w295, y=w300) -> (x/y=w299:dbl)
            n90 = Add(x=w299, y=w298) -> (x+y=w297:dbl)
            n91 = local write "SND"(w297) -> ()
          }
        }
        n92 = local write "P7"(FALSE) -> ()
      }
      frame "ReadPower" {
        # "Read power flag of the PMT-Module"
        n93 = local read "PowerD"() -> (w315:i32)
        n94 = call "Read HV.vi"("HV"=w315, "handle"=w314) -> ("HV out"=w313:i32)  [unwired: 7 in, 2 out]
        n95 = local write "PowerD"(w313) -> ()
        n96 = local write "P2"(FALSE ("P2")) -> ()
      }
      frame "ReadIT" {
        # "Read internal time of the PMT-Module"
        n97 = local read "ITD"() -> (w343:i32)
        n98 = call "Read IT.vi"("IT"=w343, "handle"=w342) -> ("IT out"=w341:i32)  [unwired: 7 in, 2 out]
        n99 = local write "ITD"(w341) -> ()
        n100 = local write "P4"(FALSE ("P4")) -> ()
      }
      frame "ReadRN" {
        # "Read data read number of the PMT-Module"
        n101 = local read "RND"() -> (w371:i32)
        n102 = call "Read RN.vi"("RN"=w371, "handle"=w370) -> ("RN out"=w368:i32)  [unwired: 7 in, 2 out]
        n103 = local write "RND"(w368) -> ()
        n104 = local write "P6"(FALSE ("P4")) -> ()
      }
      frame "ReadSN" {
        # "Read data sweep number of the Motorized stage"
        n105 = Increment(x=w388) -> (x+1=w389:i32)
        n106 = local write "SN"(w389) -> ()
      }
      frame "CountStart" {
        # "Conter Start!"
        n107 = local read "Correction"() -> (w421:bool)
        n108 = Boolean To (0,1)(Boolean=w421) -> (0, 1=w423:i16)
        n109 = To Long Integer(number=w423) -> (32bit integer=w422:i32)
        n110 = call "Count Start.vi"("Correction"=w422, "handle"=w424) -> ()  [unwired: 8 in, 2 out]
      }
      frame "CountStop" {
        w442 = FALSE ("Start")
        # "Add Auto Sweep button local variable here"
        # "Conter Stop!"
        n111 = local write "Auto-Sweep"(w442) -> ()
        n112 = local write "Stop"(w442) -> ()
        n113 = local write "Start"(w442) -> ()
        n114 = call "Count Stop.vi"("handle"=w453) -> ()  [unwired: 9 in, 2 out]
        n115 = Build Array (concatenate)(w451, "ActiveSwitch") -> (w450:string[])
      }
      frame "ReadData" {
        # "Read Data...."
        n116 = flat-sequence {
          tunnel: w487 -> [w502]
          tunnel: [w502] -> w472
          tunnel: w486 -> [w501]
          tunnel: [w501] -> w471
          tunnel: w483 -> [w500]
          tunnel: [w500] -> w470
          tunnel: w472 -> [w517]
          tunnel: w471 -> [w506]
          tunnel: [w506] -> w469
          tunnel: [w507] -> w468
          tunnel: w470 -> [w510]
          tunnel: [w512] -> w467
          tunnel: [w511] -> w466
          tunnel: w469 -> [w526]
          tunnel: [w525] -> w485
          tunnel: [w518] -> w484
          tunnel: w468 -> [w518]
          tunnel: w467 -> [w523]
          tunnel: w466 -> [w524]
          frame #0 {
            # "DB Clear!"
            n117 = Initialize Array(u32 0, 16 ("次元サイズ")) -> (w503:u32[])
            n118 = local write "DB"(w503) -> ()
          }
          frame #1 {
            n119 = local read "OLD"() -> (w514:i32)
            n120 = local read "GN"() -> (w516:i32)
            n121 = local read "DB"() -> (w515:u32[])
            n122 = call "Read Data.vi"("OLD"=w514, "DataBuf"=w515, "GateNum"=w516, "handle"=w517) -> ("OLD out"=w513:i32, "DataBuf out"=w511:u32[], "GateNum out"=w509:i32, "function return"=w512:u32)  [unwired: 3 in, 1 out]
            n123 = local write "OLD"(w513) -> ()
            n124 = local write "GN"(w509) -> ()
            n125 = local write "DB"(w511) -> ()
            n126 = Build Array(w509) -> (w508:i32[])
            n127 = Build Array (concatenate)(w510, w508) -> (w507:i32[])
          }
          frame #2 {
            # "Check Over Rang !"
            # "ADD Data DIM"
            # "Pickup Tans Data!"
            n128 = To Long Integer(number=w523) -> (32bit integer=w521:i32)
            n129 = local read "OLD"() -> (w520:i32)
            n130 = Array Subset(array=w524, length=w521) -> (w522:u32[])  [unwired: 1 in]
            n131 = Not Equal To 0?(x=w520) -> (x != 0?=w519:bool)
            n132 = local write "OVL"(w519) -> ()
            n133 = Build Array (concatenate)(w526, w522) -> (w525:u32[])
            n134 = local write "Graph"(w525) -> ()
          }
        }
      }
      frame "AutoReadData" {
        # "Read Data...."
        n135 = stacked-sequence {
          tunnel: w532 -> [w574]
          tunnel: [w573] -> w539
          tunnel: w538 -> [w568]
          tunnel: w537 -> [w572]
          tunnel: w536 -> [w571]
          tunnel: [w570] -> w535
          tunnel: w532 -> [w569]
          tunnel: w530 -> [w563]
          tunnel: [w561] -> w529
          tunnel: "Rotating" -> [w558]
          frame #0 {
            n136 = local read "SP"() -> (w565:dbl)
            n137 = local read "SS"() -> (w560:dbl)
            n138 = Array Size(array=w568) -> (size(s)=w567:i32)
            n139 = Multiply(x=w560, y=w558) -> (x*y=w559:dbl)
            n140 = Multiply(x=w559, y=w567) -> (x*y=w566:dbl)
            n141 = Add(x=w565, y=w566) -> (x+y=w564:dbl)
            n142 = Bundle("mean"=w569, w564) -> (w562:cluster{"mean":dbl, dbl})  [unwired: 1 in]
            n143 = Build Array (concatenate)(w572, w571) -> (w570:dbl[])
            n144 = Build Array (concatenate)(w568, w574) -> (w573:dbl[])
            n145 = Build Array (concatenate)(w563, w562) -> (w561:cluster{"mean":dbl, dbl}[])
            n146 = local write "Sweep Graph"(w573) -> ()
          }
        }
        n147 = property on="Polar Plot" class="Pict"() -> ("Draw Area Size"=w534:T3)  [unwired: 2 in, 2 out]
        n148 = call <vilib>:"Polar Plot with Point Options.vi"("data array [mag, phase (deg)]"=w529, "dimensions (w,h)"=w534) -> ("new picture"=→"Polar Plot":picture)  [unwired: 13 in]
      }
      frame "CountInit" {
        w587 = 0
        # "Auto"
        # "Clear Data DIM !"
        n149 = Initialize Array(w587, w587) -> (w585:i32[])
        n150 = Build Array("LockSwitch", "ReadRN", "CountStart", "ReadData", "CheckNumber") -> (w588:string[])
        n151 = Build Array (concatenate)(w594, w588) -> (w593:string[])
      }
      frame "AutoCount|nit!" {
        w624 = 0
        # "Clear Data DIM !"
        n152 = local read "SND"() -> (w611:i32)
        n153 = local read "SN"() -> (w616:i32)
        n154 = Increment(x=w611) -> (x+1=w612:i32)
        n155 = Less?(x=w616, y=w612) -> (x < y?=w615:bool)
        n156 = Initialize Array(w624, w624) -> (w623:i32[])
        n157 = case shown="True" w615 {
          tunnel: w614 -> [w640 w643]
          tunnel: [w638 w642] -> w613
          frame False {
            n158 = Build Array("AutoReadData", "AutoCheckNumber") -> (w639:string[])
            n159 = Build Array (concatenate)(w640, w639) -> (w638:string[])
          }
          frame True {
            n160 = Build Array("LockSwitch", "ReadRN", "CountStart", "ReadData", "AutoCheckNumber") -> (w649:string[])
            n161 = Build Array (concatenate)(w643, w649) -> (w642:string[])
          }
        }
      }
      frame "CheckNumber" {
        # "Add append"
        # "Add Case Strucutre outside\nsimilar to GN,"
        # "Check RN and Data lenbgth,Stop Switch ......"
        n162 = local read "Stop"() -> (w662:bool)
        n163 = local read "GN"() -> (w663:i32)
        n164 = Decrement(x=w665) -> (x-1=w664:i32)
        n165 = Less?(x=w663, y=w664) -> (x < y?=w669:bool)
        n166 = case shown="False" w669 {
          tunnel: [w684 w686] -> w666
          tunnel: w662 -> [_ w685]
          frame False {
            # "\"MotorJog\"; here"
            # "Move \"Active Swith\" to False Condition of Position Number"
            # "Add \"AutoExport Run\" here"
            n167 = local write "Start"(FALSE ("Start")) -> ()
            n168 = Build Array("CountStop", "ActiveSwitch") -> (w684:string[])
          }
          frame True {
            n169 = case shown="False" w685 {
              tunnel: [w688 w690] -> w686
              frame False {
                n170 = Build Array("ReadData", "CheckNumber") -> (w688:string[])
              }
              frame True {
                n171 = Build Array("CountStop") -> (w690:string[])
              }
            }
          }
        }
        n172 = Build Array (concatenate)(w667, w666) -> (w668:string[])
      }
      frame "AutoCheckNumber" {
        # "Add append"
        # "Add Case Strucutre outside\nsimilar to GN,"
        # "Check RN and Data lenbgth,Stop Switch ......"
        n173 = local read "Stop"() -> (w707:bool)
        n174 = local read "SND"() -> (w696:i32)
        n175 = local read "SN"() -> (w700:i32)
        n176 = Less?(x=w700, y=w696) -> (x < y?=w699:bool)
        n177 = case shown="True" w699 {
          tunnel: [w724 w734] -> w709
          tunnel: w708 -> [_ w733]
          tunnel: w707 -> [_ w730]
          tunnel: [TRUE w729] -> w702
          frame False {
            w728 = FALSE ("Start")
            n178 = local write "Auto-Sweep"(w728) -> ()
            n179 = local write "Start"(w728) -> ()
            n180 = Build Array("CountStop", "AutoExportSweep", "ActiveSwitch") -> (w724:string[])
          }
          frame True {
            n181 = local read "GN"() -> (w731:i32)
            n182 = Decrement(x=w733) -> (x-1=w732:i32)
            n183 = Less?(x=w731, y=w732) -> (x < y?=w735:bool)
            n184 = case shown="True" w735 {
              tunnel: [w737 w753] -> w734
              tunnel: w730 -> [w738 w752]
              tunnel: [w736 w751] -> w729
              frame False {
                # "\"MotorJog\"; here"
                # "Move \"Active Swith\" to False Condition of Position Number"
                # "Add \"AutoExport Run\" here"
                n185 = case shown="False" w738 {
                  tunnel: [w744 w749] -> w737
                  tunnel: [FALSE TRUE] -> w736
                  frame False {
                    n186 = Build Array("CountStop", "AutoExportRun", "AutoReadData", "ReadSN", "MotorJog", "AutoCount|nit!") -> (w744:string[])
                  }
                  frame True {
                    n187 = local write "Auto-Sweep"(TRUE) -> ()
                    n188 = Build Array("CountStop") -> (w749:string[])
                  }
                }
              }
              frame True {
                n189 = case shown="False" w752 {
                  tunnel: [w756 w760] -> w753
                  tunnel: [FALSE TRUE] -> w751
                  frame False {
                    n190 = Build Array("ReadData", "AutoCheckNumber") -> (w756:string[])
                  }
                  frame True {
                    n191 = Build Array("CountStop") -> (w760:string[])
                    n192 = local write "Auto-Sweep"(TRUE) -> ()
                  }
                }
              }
            }
          }
        }
        n193 = Build Array (concatenate)(w710, w709) -> (w711:string[])
      }
      frame "Export" {
        # "For Auto Export also add mean waveform"
        # "Get mean Data into 1D array Shift register for waveform"
        # "Gate Number is just number of count measurements"
        # "time...using array size"
        # "time...using array size"
        n194 = Array Size(array=w780) -> (size(s)=w792:i32)
        n195 = for {
          N: w792 -> [_]
          tunnel: [w807] -> w779 mode=indexing
          i -> [w809]
          n196 = local read "ITD"() -> (w811:i32)
          n197 = Add(x=1, y=w809) -> (x+y=w810:i32)
          n198 = Multiply(x=w811, y=w810) -> (x*y=w807:i32)
        }
        n199 = call <vilib>:"Std Deviation and Variance.vi"("X"=w780) -> ("mean"=w773:dbl, "standard deviation"=w772:dbl)  [unwired: 1 in, 1 out]
        n200 = Build Array(w773, w772) -> (w771:dbl[])
        n201 = Build Array(w775, w779, w780) -> (w790:u32[][])
        n202 = call-poly <vilib>:"Write Delimited Spreadsheet.vi"("1D data"=string[] ["Gate  No.", "Time [ms]", "Counts"], "append to file? (new file:F)"=FALSE, "transpose? (no:F)"=FALSE) -> ("new file path (Not A Path if cancelled)"=w789:path)  [unwired: 11 in, 1 out]
        n203 = call-poly <vilib>:"Write Delimited Spreadsheet.vi"("file path (dialog if empty)"=w789, "2D data"=w790, "append to file? (new file:F)"=TRUE, "transpose? (no:F)"=TRUE) -> ("new file path (Not A Path if cancelled)"=w785:path)  [unwired: 10 in, 1 out]
        n204 = call-poly <vilib>:"Write Delimited Spreadsheet.vi"("file path (dialog if empty)"=w785, "1D data"=string[] ["Mean", "Std. Dev."], "append to file? (new file:F)"=TRUE, "transpose? (no:F)"=FALSE) -> ("new file path (Not A Path if cancelled)"=w781:path)  [unwired: 10 in, 1 out]
        n205 = call-poly <vilib>:"Write Delimited Spreadsheet.vi"("file path (dialog if empty)"=w781, "1D data"=w771, "append to file? (new file:F)"=TRUE, "transpose? (no:F)"=FALSE) -> ()  [unwired: 10 in, 2 out]
        n206 = local write "Export"(FALSE) -> ()
      }
      frame "AutoExportRun" {
        # "For Auto Export also add mean waveform"
        # "Get mean Data into 1D array Shift register for waveform"
        # "Gate Number is just number of count measurements"
        # "time...using array size"
        n207 = Array Size(array=w831) -> (size(s)=w833:i32)
        n208 = for {
          N: w833 -> [_]
          tunnel: [w875] -> w830 mode=indexing
          i -> [w877]
          n209 = local read "ITD"() -> (w879:i32)
          n210 = Add(x=1, y=w877) -> (x+y=w878:i32)
          n211 = Multiply(x=w879, y=w878) -> (x*y=w875:i32)
        }
        n212 = flat-sequence {
          tunnel: w822 -> [w874]
          tunnel: [w870] -> w821
          frame #0 {
            n213 = local read "SS"() -> (w873:dbl)
            n214 = Multiply(x=w874, y=w873) -> (x*y=w871:dbl)
            n215 = local read "SP"() -> (w872:dbl)
            n216 = Add(x=w872, y=w871) -> (x+y=w870:dbl)
          }
        }
        n217 = call <vilib>:"Std Deviation and Variance.vi"("X"=w831) -> ("mean"=w825:dbl, "standard deviation"=w815:dbl)  [unwired: 1 in, 1 out]
        n218 = Build Array(w825, w815) -> (w828:dbl[])
        n219 = Number To Decimal String(number=w821) -> (decimal integer string=w820:string)  [unwired: 1 in]
        n220 = Build Array(w817, w830, w831) -> (w832:u32[][])
        n221 = Build Array (concatenate)(string[] ["Angle (deg)"], w820) -> (w818:string[])
        n222 = case shown="True" "Save All Gate Data" {
          tunnel: w832 -> [_ w868]
          tunnel: w828 -> [_ w855]
          tunnel: [w848 w854] -> w827
          tunnel: w823 -> [w848 w853]
          tunnel: w818 -> [_ w849]
          frame False {
          }
          frame True {
            # "time...using array size"
            n223 = call-poly <vilib>:"Write Delimited Spreadsheet.vi"("file path (dialog if empty)"=w853, "1D data"=w849, "append to file? (new file:F)"=TRUE, "transpose? (no:F)"=FALSE) -> ("new file path (Not A Path if cancelled)"=w852:path)  [unwired: 10 in, 1 out]
            n224 = call-poly <vilib>:"Write Delimited Spreadsheet.vi"("file path (dialog if empty)"=w852, "1D data"=string[] ["Gate  No.", "Time [ms]", "Counts"], "append to file? (new file:F)"=TRUE, "transpose? (no:F)"=FALSE) -> ("new file path (Not A Path if cancelled)"=w867:path)  [unwired: 10 in, 1 out]
            n225 = call-poly <vilib>:"Write Delimited Spreadsheet.vi"("file path (dialog if empty)"=w867, "2D data"=w868, "append to file? (new file:F)"=TRUE, "transpose? (no:F)"=TRUE) -> ("new file path (Not A Path if cancelled)"=w863:path)  [unwired: 10 in, 1 out]
            n226 = call-poly <vilib>:"Write Delimited Spreadsheet.vi"("file path (dialog if empty)"=w863, "1D data"=string[] ["Mean", "Std. Dev."], "append to file? (new file:F)"=TRUE, "transpose? (no:F)"=FALSE) -> ("new file path (Not A Path if cancelled)"=w859:path)  [unwired: 10 in, 1 out]
            n227 = call-poly <vilib>:"Write Delimited Spreadsheet.vi"("file path (dialog if empty)"=w859, "1D data"=w855, "append to file? (new file:F)"=TRUE, "transpose? (no:F)"=FALSE) -> ("new file path (Not A Path if cancelled)"=w854:path)  [unwired: 10 in, 1 out]
          }
        }
        n228 = local write "Export"(FALSE) -> ()
      }
      frame "AutoExportSweep" {
        w890 = 0
        w889 = 0.0
        # "Gate Number is just number \nof count measurements"
        # "For Auto Export also add mean waveform"
        # "Get mean Data into 1D array Shift register for waveform"
        # "time...using array size"
        # "time...using array size"
        n229 = Array Size(array=w908) -> (size(s)=w923:i32)
        n230 = for {
          N: w923 -> [_]
          tunnel: [w958] -> w915 mode=indexing
          i -> [w955]
          n231 = local read "SS"() -> (w959:dbl)
          n232 = Multiply(x=w959, y=w955) -> (x*y=w956:dbl)
          n233 = local read "SP"() -> (w957:dbl)
          n234 = Add(x=w957, y=w956) -> (x+y=w958:dbl)
        }
        n235 = call <vilib>:"Std Deviation and Variance.vi"("X"=w908) -> ("mean"=w909:dbl, "standard deviation"=w903:dbl)  [unwired: 1 in, 1 out]
        n236 = Initialize Array(w889, w890) -> (w906:dbl[])
        n237 = Initialize Array(w889, w890) -> (w905:dbl[])
        n238 = Build Array(w909, w903) -> (w899:dbl[])
        n239 = Initialize Array(cluster{i32, i32} {0, 0}, w890) -> (w888:cluster{i32, i32}[])
        n240 = local read "RN"() -> (w893:i32)
        n241 = Build Array(w915, w908, w904) -> (w921:dbl[][])
        n242 = Number To Decimal String(number=w893) -> (decimal integer string=w883:string)  [unwired: 1 in]
        n243 = local read "IT"() -> (w892:i32)
        n244 = Number To Decimal String(number=w892) -> (decimal integer string=w882:string)  [unwired: 1 in]
        n245 = Build Array("Sample Name", "Laser Power (mW)", w883, w882, "Polarizer config", "Analyzer config") -> (w891:string[])
        n246 = for {
          N: 6 -> [_]
          shift-right: [w943] -> w894
          shift-left: w897 -> [w944]
          tunnel: string[] ["#Sample", "#LaserPower (mW)", "#NumGates", "#GateTime (ms)", "#PolarizerConfig", "#AnalyzerConfig"] -> [w939] mode=indexing
          tunnel: w891 -> [w938] mode=indexing
          n247 = Build Array(w939, w938) -> (w940:string[])
          n248 = call-poly <vilib>:"Write Delimited Spreadsheet.vi"("file path (dialog if empty)"=w944, "1D data"=w940, "append to file? (new file:F)"=TRUE, "transpose? (no:F)"=FALSE) -> ("new file path (Not A Path if cancelled)"=w943:path)  [unwired: 10 in, 1 out]
        }
        n249 = call-poly <vilib>:"Write Delimited Spreadsheet.vi"("file path (dialog if empty)"=w894, "1D data"=string[] ["Angle", "CountsMean", "CountsSTD"], "append to file? (new file:F)"=TRUE, "transpose? (no:F)"=FALSE) -> ("new file path (Not A Path if cancelled)"=w920:path)  [unwired: 10 in, 1 out]
        n250 = call-poly <vilib>:"Write Delimited Spreadsheet.vi"("file path (dialog if empty)"=w920, "2D data"=w921, "append to file? (new file:F)"=TRUE, "transpose? (no:F)"=TRUE) -> ("new file path (Not A Path if cancelled)"=w917:path)  [unwired: 10 in, 1 out]
        n251 = case shown="True" FALSE {
          tunnel: w917 -> [w945 w953]
          tunnel: w899 -> [_ w950]
          tunnel: [w945 w947] -> w898
          frame False {
          }
          frame True {
            n252 = call-poly <vilib>:"Write Delimited Spreadsheet.vi"("file path (dialog if empty)"=w953, "1D data"=string[] ["Mean", "Std. Dev."], "append to file? (new file:F)"=TRUE, "transpose? (no:F)"=FALSE) -> ("new file path (Not A Path if cancelled)"=w951:path)  [unwired: 10 in, 1 out]
            n253 = call-poly <vilib>:"Write Delimited Spreadsheet.vi"("file path (dialog if empty)"=w951, "1D data"=w950, "append to file? (new file:F)"=TRUE, "transpose? (no:F)"=FALSE) -> ("new file path (Not A Path if cancelled)"=w947:path)  [unwired: 10 in, 1 out]
          }
        }
        n254 = local write "Export"(FALSE) -> ()
      }
      frame "AutoSweep" {
        w968 = 0
        # "1. Create a file path (Send two strings, \"SetPosition\" and \"AutoCount|nit!\")\n2. Send to \"SetPosition\"\n2.1. Will create a Position Number Shift register\n2.2. Move stage to initial position, allow time to complete movement or add delay\n3. Send to \"AutoCount|nit!\"\n3.1. \"AutoCount|nit!\" is clone of \"Count|nit!\" but sends to \"AutoCheckNumber\", not \"CheckNumber\n3.1.1. \"AutoCheckNumber\" will check if end position, or run condition is met then send \"CountStop\" and \"ActiveSwitch\"\n3.1.2. \"AutoCheck Number\" will allow \"CountStop\" to be sent via Stop Boolean\n3.1.3. \"AutoCheckNumber\" will upon END of one run will run \"AutoExportRun\" to set file path\n3.1.3.1. \"AutoExportRun\" will add a data point to Mean Waveform after Count Stop\n3.1.4. \"AutoCheckNumber\" will upon END of sweep will run \"AutoExportSweep\" then issue \"ActiveSwitch\"\n3.1.4.1. \"AutoExportSweep\" will append final Mean Sweep waveform to file path before \"CountStop\";\"ActiveSwitch\"\n4. If End condition not met; \"MotorJog\"; \"AutoCount|nit!\"....repeats\n4.1. Will move to next position by set increment, with .net code, add delay to allow it to arrive at position"
        # "Create a File path here\nSend switch case string \"SetPosition\", which has a position number switch register"
        # "1.Position Set, create a file path\n2. Count|nit!---duplicate and create auto counter, add read sweep data for auto read\n2.0.1Checknumber end, change active switch to Auto export\n3. Auto Export ... need to make \n3.0.2Auto Export end, send to read sweep data (mean, stdev for per sweep)\n3.Export\n4.check end position, check end condition met\n5.met>end;not end >continue\n6. Jog motor\n7.repeat from 2."
        # "Create Motor Controls for setting Homing, Step size for angle, idle time(if required),"
        n255 = local write "SN"(w968) -> ()
        n256 = call-poly <vilib>:"Write Delimited Spreadsheet.vi"("file path (dialog if empty)"="autosweep file to save", "append to file? (new file:F)"=FALSE) -> ("new file path (Not A Path if cancelled)"=w967:path)  [unwired: 12 in, 1 out]
        n257 = Build Array("SetPosition", "AutoCount|nit!") -> (w973:string[])
        n258 = Build Array (concatenate)(w971, w973) -> (w970:string[])
        n259 = Wait (ms)(milliseconds to wait="Wait to Start (ms)") -> ()  [unwired: 1 out]
      }
      frame "MotorJog" {
        # "Move position by set increment"
        # "Add a test Jog?"
        # "Put thor labs net code here"
        n260 = flat-sequence {
          tunnel: w1006 -> [w1030]
          tunnel: [w1030] -> w995
          tunnel: w996 -> [w1025]
          tunnel: [w1025] -> w994
          tunnel: w993 -> [w1024]
          tunnel: [w1024] -> w992
          tunnel: w995 -> [w1043]
          tunnel: w994 -> [w1038]
          tunnel: w992 -> [w1037]
          frame #0 {
            n261 = case shown="True" w1024 {
              tunnel: w1025 -> [_ w1034]
              frame False {
              }
              frame True {
                n262 = local read "SSD"() -> (w1032:dbl)
                n263 = Multiply(x=w1032, y=2 ("step size multiple for polarizer2")) -> (x*y=w1033:dbl)
                n264 = invoke class="KCubeDCServo" method="MoveRelative"(reference=w1034, "direction"=1, "stepSize"=w1033, "waitTimeout"=0) -> ()  [unwired: 2 in, 6 out]
              }
            }
            n265 = local read "SSD"() -> (w1029:dbl)
            n266 = invoke class="KCubeDCServo" method="MoveRelative"(reference=w1030, "direction"=1, "stepSize"=w1029, "waitTimeout"=0) -> ()  [unwired: 2 in, 6 out]
            n267 = local read "WT"() -> (w1027:i32)
            n268 = Wait (ms)(milliseconds to wait=w1027) -> ()  [unwired: 1 out]
          }
          frame #1 {
            n269 = case shown="True" w1037 {
              tunnel: w1038 -> [_ w1044]
              frame False {
              }
              frame True {
                n270 = invoke class="KCubeDCServo" method="GetPositionCounter"(reference=w1044) -> ("GetPositionCounter"=w1047:i32)  [unwired: 2 in, 2 out]
                n271 = Divide(x=w1047, y=1919.6418578623338) -> (x/y=w1045:dbl)
                n272 = local write "PC 2"(w1045) -> ()
              }
            }
            n273 = invoke class="KCubeDCServo" method="GetPositionCounter"(reference=w1043) -> ("GetPositionCounter"=w1041:i32)  [unwired: 2 in, 2 out]
            n274 = Divide(x=w1041, y=1919.6418578623338) -> (x/y=w1039:dbl)
            n275 = local write "PC"(w1039) -> ()
            n276 = Wait (ms)(milliseconds to wait=50) -> ()  [unwired: 1 out]
          }
        }
        n277 = local write "P8"(FALSE) -> ()
      }
      frame "SetPosition" {
        n278 = flat-sequence {
          tunnel: w1062 -> [w1083]
          tunnel: [w1083] -> w1053
          tunnel: w1051 -> [w1081]
          tunnel: [w1081] -> w1050
          tunnel: w1048 -> [w1080]
          tunnel: w1053 -> [w1090]
          tunnel: [w1090] -> w1052
          tunnel: w1050 -> [w1088]
          tunnel: [w1088] -> w1049
          tunnel: w1048 -> [w1086]
          tunnel: w1052 -> [w1099]
          tunnel: w1049 -> [w1094]
          tunnel: w1048 -> [w1093]
          frame #0 {
            n279 = case shown="True" w1080 {
              tunnel: w1081 -> [_ w1085]
              frame False {
              }
              frame True {
                n280 = local read "SPD 2"() -> (w1084:dbl)
                n281 = invoke class="KCubeDCServo" method="SetMoveAbsolutePosition"(reference=w1085, "position"=w1084) -> ()  [unwired: 2 in, 4 out]
              }
            }
            n282 = local read "SPD"() -> (w1082:dbl)
            n283 = invoke class="KCubeDCServo" method="SetMoveAbsolutePosition"(reference=w1083, "position"=w1082) -> ()  [unwired: 2 in, 4 out]
          }
          frame #1 {
            w1087 = 0
            n284 = case shown="True" w1086 {
              tunnel: w1088 -> [_ w1092]
              tunnel: w1087 -> [_ w1091]
              frame False {
              }
              frame True {
                n285 = invoke class="KCubeDCServo" method="MoveAbsolute"(reference=w1092, "waitTimeout"=w1091) -> ()  [unwired: 2 in, 4 out]
              }
            }
            n286 = invoke class="KCubeDCServo" method="MoveAbsolute"(reference=w1090, "waitTimeout"=w1087) -> ()  [unwired: 2 in, 4 out]
            n287 = local read "WT"() -> (w1089:i32)
            n288 = Wait (ms)(milliseconds to wait=w1089) -> ()  [unwired: 1 out]
          }
          frame #2 {
            n289 = case shown="True" w1093 {
              tunnel: w1094 -> [_ w1101]
              frame False {
              }
              frame True {
                n290 = invoke class="KCubeDCServo" method="GetPositionCounter"(reference=w1101) -> ("GetPositionCounter"=w1102:i32)  [unwired: 2 in, 2 out]
                n291 = Divide(x=w1102, y=1919.6418578623338) -> (x/y=w1100:dbl)
                n292 = local write "PC 2"(w1100) -> ()
              }
            }
            n293 = invoke class="KCubeDCServo" method="GetPositionCounter"(reference=w1099) -> ("GetPositionCounter"=w1096:i32)  [unwired: 2 in, 2 out]
            n294 = Divide(x=w1096, y=1919.6418578623338) -> (x/y=w1095:dbl)
            n295 = local write "PC"(w1095) -> ()
            n296 = Wait (ms)(milliseconds to wait=50) -> ()  [unwired: 1 out]
          }
        }
      }
      frame "", "Idle" {
        n297 = event shown="[12] \"Auto-Sweep\": Value Change" {
          selector: _ -> [_ _ _ _ _ _ _ _ _ _ _ _ _]
          dyn-events: _ -> [_ _ _ _ _ _ _ _ _ _ _ _ _]
          timeout: _ -> [_ _ _ _ _ _ _ _ _ _ _ _ _]
          tunnel: w1119 -> [w1134 w1137 w1140 w1144 w1148 w1152 w1156 w1160 w1163 w1165 w1168 w1171 w1174]
          tunnel: [w1132 w1136 w1139 w1143 w1147 w1151 w1155 w1159 w1162 w1164 w1167 w1170 w1175] -> w1117
          event Menu Selection (User) {
            n298 = event-data() -> ("ItemTag"=w1133:string)  [unwired: 1 out]
            n299 = Build Array (concatenate)(w1134, w1133) -> (w1132:string[])
          }
          event "EXIT": Value Change {
            n300 = event-data() -> ()  [unwired: 7 out]
            n301 = Build Array (concatenate)(w1137, "Exit") -> (w1136:string[])
          }
          event "P1": Value Change {
            n302 = event-data() -> ()  [unwired: 7 out]
            n303 = Build Array (concatenate)(w1140, "SetPower") -> (w1139:string[])
          }
          event "P2": Value Change {
            n304 = event-data() -> ()  [unwired: 7 out]
            n305 = Build Array (concatenate)(w1144, "ReadPower") -> (w1143:string[])
            n306 = Wait (ms)(milliseconds to wait=u32 200 ("ミリ秒待機時間")) -> ()  [unwired: 1 out]
          }
          event "P3": Value Change {
            n307 = event-data() -> ()  [unwired: 7 out]
            n308 = Build Array (concatenate)(w1148, "SetIT") -> (w1147:string[])
            n309 = Wait (ms)(milliseconds to wait=u32 200 ("ミリ秒待機時間")) -> ()  [unwired: 1 out]
          }
          event "P4": Value Change {
            n310 = event-data() -> ()  [unwired: 7 out]
            n311 = Build Array (concatenate)(w1152, "ReadIT") -> (w1151:string[])
            n312 = Wait (ms)(milliseconds to wait=u32 200 ("ミリ秒待機時間")) -> ()  [unwired: 1 out]
          }
          event "P5": Value Change {
            n313 = event-data() -> ()  [unwired: 7 out]
            n314 = Build Array (concatenate)(w1156, "SetRN") -> (w1155:string[])
            n315 = Wait (ms)(milliseconds to wait=u32 200 ("ミリ秒待機時間")) -> ()  [unwired: 1 out]
          }
          event "P6": Value Change {
            n316 = event-data() -> ()  [unwired: 7 out]
            n317 = Build Array (concatenate)(w1160, "ReadRN") -> (w1159:string[])
            n318 = Wait (ms)(milliseconds to wait=u32 200 ("ミリ秒待機時間")) -> ()  [unwired: 1 out]
          }
          event "Start": Value Change {
            n319 = event-data() -> ()  [unwired: 7 out]
            n320 = Build Array (concatenate)(w1163, "CountInit") -> (w1162:string[])
          }
          event "Export": Value Change {
            n321 = event-data() -> ()  [unwired: 7 out]
            n322 = Build Array (concatenate)(w1165, "Export") -> (w1164:string[])
          }
          event "P7": Value Change {
            n323 = event-data() -> ()  [unwired: 7 out]
            n324 = Build Array (concatenate)(w1168, "SetStepProp") -> (w1167:string[])
          }
          event "P8": Value Change {
            n325 = event-data() -> ()  [unwired: 7 out]
            n326 = Build Array (concatenate)(w1171, "MotorJog") -> (w1170:string[])
          }
          event "Auto-Sweep": Value Change {
            n327 = event-data() -> ()  [unwired: 7 out]
            n328 = Build Array (concatenate)(w1174, "AutoSweep") -> (w1175:string[])
            n329 = Wait (ms)(milliseconds to wait=200) -> ()  [unwired: 1 out]
          }
        }
        n330 = Build Array (concatenate)("", w1117) -> (w1116:string[])
      }
      frame "Error", Default {
        n331 = Concatenate Strings("Error  Case Name .....", "\r\n", w1188) -> (w1190:string)
        n332 = One Button Dialog(message=w1190) -> (true=w1189:bool)  [unwired: 1 out]
        n333 = stacked-sequence {
          tunnel: w1189 -> [_]
          frame #0 {
            n334 = Stop() -> ()  [unwired: 1 out]
          }
        }
      }
      frame "Exit" {
        # "See you again ......"
        n335 = call "ClosePMT.vi"("Handle"=w1207) -> ()  [unwired: 9 in, 2 out]
      }
    }
    n336 = case shown="True" w30 {
      tunnel: w34 -> [_ w89]
      frame False {
      }
      frame True {
        n337 = invoke class="KCubeDCServo" method="GetPositionCounter"(reference=w89) -> ("GetPositionCounter"=w91:i32)  [unwired: 2 in, 2 out]
        n338 = Divide(x=w91, y=1919.6418578623338) -> (x/y=w90:dbl)
        n339 = local write "PC 2"(w90) -> ()
      }
    }
    n340 = call "SM_CaseErase.vi"("Input"=w67) -> ("Output"=w66:string[])  [unwired: 10 out]
  }
  n341 = case shown="True" w3 {
    tunnel: w6 -> [_ w1232]
    frame False {
    }
    frame True {
      n342 = invoke class="KCubeDCServoControl" method="CloseDevice"(reference=w1232) -> ()  [unwired: 2 in, 3 out]
    }
  }
  n343 = invoke class="KCubeDCServoControl" method="CloseDevice"(reference=w14) -> ()  [unwired: 2 in, 3 out]
